vi "2.0.0_BEMF_Calibration.vi"(7 "Data in":T2, 8 "error in (no error)":errorcluster, 9 "AllControls In":T1, 10 "?":T3, 11 "Message Queue out":T4) -> (0 "error out":errorcluster, 1 "Flow":string, 2 "Data":T3, 3 "Message Queue Out":T4, 5 "Data out":T2)   [LabVIEW 2017]
uses:
  Depends/AMC/subVIs/TypeDefs/amc_Message Queue.ctl
  Depends/AMC/subVIs/TypeDefs/amc_Message.ctl
  Depends/Tools/Keyed Array/Tools_KeyedArray KeyedArray.ctl
  Ctrls/Data.ctl
  Ctrls/CSV_Data.ctl
  Ctrls/AllControls.ctl
  DIPC 692 Daemon API/typdef/calibration.ctl
  Ctrls/AlarmIndex.ctl
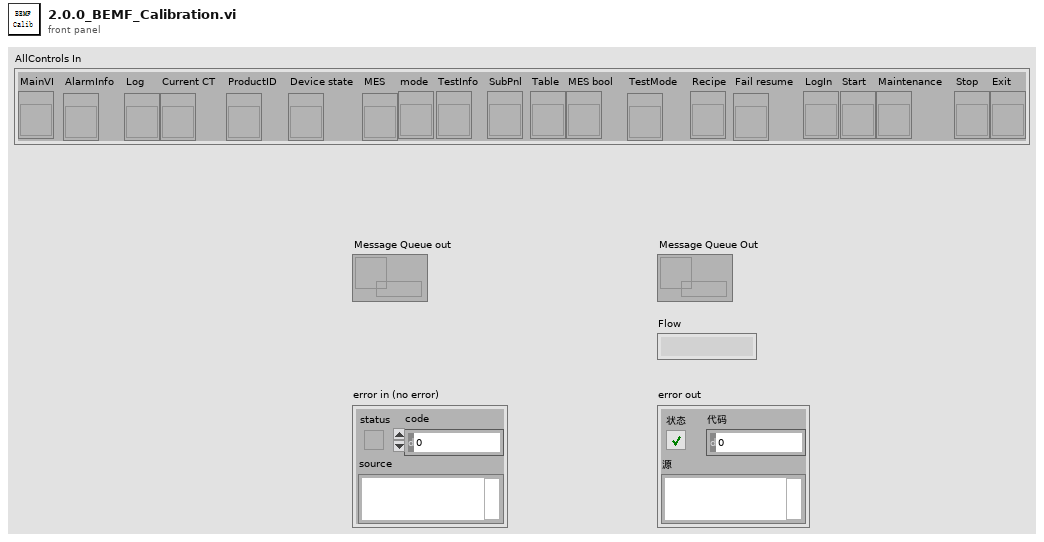
[diagram p1: front panel]
types:
  T1 = typedef "AllControls.ctl" = cluster{"MainVI":refnum<vi>, "AlarmInfo":refnum<vi>, "Log":refnum<vi>, "Current CT":refnum<vi>, "ProductID":refnum<vi>, "Device state":refnum<vi>, "MES":refnum<vi>, "mode":refnum<vi>, "TestInfo":refnum<vi>, "SubPnl":refnum<vi>, "Table":refnum<vi>, "MES bool":refnum<vi>, "TestMode":refnum<vi>, "Recipe":refnum<vi>, "Fail resume":refnum<vi>, "LogIn":refnum<vi>, "Start":refnum<vi>, "Maintenance":refnum<vi>, "Stop":refnum<vi>, "Exit":refnum<vi>}
  T2 = typedef "CSV_Data.ctl" = cluster{"Initialisation":cluster{"LMT - Connect UUT (con COM)":string, "LMT - Software Version (rrel)":string, "LMT - Write SKU file (wskuc)":string, "LMT - SKU file name":string, "Connect UUT DDM":string, "Read DDM EOL Timestamp - Mode":string, "Read DDM EOL Timestamp - Timestamp":string, "Read DDM EOL Timestamp - Rig ID":string, "Read DDM EOL Timestamp - Passmark ID":string, "Read DDM EOL Timestamp - Passmark Rev":string, "Software Version before flashing":string, "Read Hardware Serial":string, "UUT DDM SN":string, "Compare DDM SN with MES SN":string, "Backup PCBA Calibration EEPROM Response - CAL":string, "Flash Firmware Version":string, "Check SW Version":string, "Read DDM SW Version after flashing":string, "Set SKU Config":string, "Ready Status":string, "Set Device Mode to EOL":string, "DDM Parameter - Voltage":string, "DDM Parameter - Current":string, "DDM Parameter - Power":string, "DDM Parameter - Speed":string, "DDM Parameter - Pressure":string, "Tester Parameter - Voltage":string, "Tester Parameter - Current":string, "Tester Parameter - Power":string, "Tester Parameter - Ambient Pressure":string, "Tester Parameter - Ambient Temperature":string, "Calculated Parameter - DDM Pressure Corrected":string, "Calculated Parameter - DDM Real Power":string, "Calculated Parameter - Delta V":string}, "BEMF_Calibration":cluster{"Calibration Result - eol_cold_bemf_temp":string, "DDM Ambient Temp":string, "Restriction Plate Diameter":string, "Calibration Result - eol_bemf_mp_cold_coef_a":string, "Calibration Result - eol_bemf_mp_cold_coef_b":string, "Calibration Result - eol_bemf_mp_cold_coef_c":string, "Calibration Result - eol_bemf_lsi_cold_ref_coeffs":string, "Get - Calibration Result - eol_bemf_lsi_speed":string, "Get - Calibration Result - eol_bemf_lsi_integral_0":string, "Calibration Result - eol_bemf_lsi_integral_1":string, "Get - Calibration Result - eol_bemf_lsi_integral_2":string, "Get - Calibration Result - eol_cold_bemf":string, "Get - Calibration Result - eol_cold_bemf_fisf":string, "Finalise Calibration":string, "Compare -Calibration Result - eol_cold_bemf":string, "Compare -Calibration Result - eol_cold_bemf_fisf":string}, "ECO":cluster{"Reset Power Tune":string, "Reset BEMF FISF Calibration":string, "Restriction Plate Diameter":string, "ECO - Stabilisation Time":string, "ECO - DDM Parameter - Voltage":string, "ECO - DDM Parameter - Current":string, "ECO - DDM Parameter - Power":string, "ECO - DDM Parameter - Measured Power":string, "ECO - DDM Parameter - Speed":string, "ECO - DDM Parameter - Pressure":string, "ECO - Tester Parameter - Voltage":string, "ECO - Tester Parameter - Current":string, "ECO - Tester Parameter - Power":string, "ECO - Tester Parameter - Ambient Pressure":string, "ECO - Tester Parameter - Ambient Temperature":string, "ECO - Tester Parameter - Ambient Humidity":string, "ECO - Calculated Parameter - DDM Pressure Corrected":string, "ECO - Calculated Parameter - DDM Real Power":string, "ECO - Calculated Parameter - Delta V":string, "ECO - Calculated Parameter - Flowrate":string, "ECO - Calculated Parameter - Airwatt":string, "ECO - Formula":string, "PT ECO - Power Tune Mode Status":string}, "BOOST":cluster{"Restriction Plate Diameter":string, "BOOST - Stabilisation Time":string, "BOOST - DDM Parameter - Voltage":string, "BOOST - DDM Parameter - Current":string, "BOOST - DDM Parameter - Power":string, "BOOST - DDM Parameter - Measured Power":string, "BOOST - DDM Parameter - Speed":string, "BOOST - DDM Parameter - Pressure":string, "BOOST - Tester Parameter - Voltage":string, "BOOST - Tester Parameter - Current":string, "BOOST - Tester Parameter - Power":string, "BOOST - Tester Parameter - Ambient Pressure":string, "BOOST - Tester Parameter - Ambient Temperature":string, "BOOST - Tester Parameter - Ambient Humidity":string, "BOOST - Calculated Parameter - DDM Pressure Corrected":string, "BOOST - Calculated Parameter - DDM Real Power":string, "BOOST - Calculated Parameter - Delta V":string, "BOOST - Calculated Parameter - Flowrate":string, "BOOST - Calculated Parameter - Airwatt":string, "BOOST - Get AM Presence":string, "Air Muscle Turn Off Status":string, "BOOST - Air Muscle Calculated Parameter - Airwatt B":string, "BOOST - Air Muscle Calculate Airwatt Delta":string, "PT BOOST - Power Tune Mode Status":string, "Finalise Calibration":string, "ECO - Get AW Calibration value":string, "BOOST - Get AW Calibration value":string}, "MAX":cluster{"Restriction Plate Diameter":string, "MAX - Stabilisation Time":string, "Get Average Delta Tmag (LSIdelta_FISFdelta_LSItmag_FISFtmag_IIRtmag)":string, "Get Average Delta Tmag FISF":string, "MAX - DDM Parameter - Voltage":string, "MAX - DDM Parameter - Current":string, "MAX - DDM Parameter - Power":string, "MAX - DDM Parameter - Measured Power":string, "MAX - DDM Parameter - Speed":string, "MAX - DDM Parameter - Pressure":string, "MAX - Tester Parameter - Voltage":string, "MAX - Tester Parameter - Current":string, "MAX - Tester Parameter - Power":string, "MAX - Tester Parameter - Ambient Pressure":string, "MAX - Tester Parameter - Ambient Temperature":string, "MAX - Tester Parameter - Ambient Humidity":string, "MAX - Calculated Parameter - DDM Pressure Corrected":string, "MAX - Calculated Parameter - DDM Real Power":string, "MAX - Calculated Parameter - Delta V":string, "MAX - Calculated Parameter - Flowrate":string, "MAX - Calculated Parameter - Airwatt":string, "MAX_FISF_Check_Average_Delta_Tmag":string, "MAX - FISF - BEMF Finetune Result":string, "MAX tune - Delta P1":string, "MAX tune - Calculated Parameter - Airwatt":string, "Calculate Delta Airwatts - MAX finetune - Delta P2":string, "MAX finetune - DDM Parameter - Voltage":string, "MAX finetune - DDM Parameter - Current":string, "MAX finetune - DDM Parameter - Power":string, "MAX finetune - DDM Parameter - Measured Power":string, "MAX finetune - DDM Parameter - Speed":string, "MAX finetune - DDM Parameter - Pressure":string, "MAX finetune - Tester Parameter - Voltage":string, "MAX finetune - Tester Parameter - Current":string, "MAX finetune - Tester Parameter - Power":string, "MAX finetune - Tester Parameter - Ambient Pressure":string, "MAX finetune - Tester Parameter - Ambient Temperature":string, "MAX finetune - Tester Parameter - Ambient Humidity":string, "MAX finetune - Calculated Parameter - DDM Pressure Corrected":string, "MAX finetune - Calculated Parameter - DDM Real Power":string, "MAX finetune - Calculated Parameter - Delta V":string, "MAX finetune - Calculated Parameter - Flowrate":string, "MAX finetune - Calculated Parameter - Airwatt":string, "Check Derate Result":string, "Delta Tmag FISF":string, "Get Hot BEMF Result":string, "Calculate delta Pressure":string, "Finalise Calibration":string, "Calculate & Check Delta BEMF":string, "Delta P Airwatts Value":string}, "LL":cluster{"DDM Ambient Temp":string, "Restriction Plate Diameter":string, "LL - DDM Parameter - Voltage":string, "LL - DDM Parameter - Current":string, "LL - DDM Parameter - Power":string, "LL - DDM Parameter - Measured Power":string, "LL - DDM Parameter - Speed":string, "LL - DDM Parameter - Pressure":string, "LL - Tester Parameter - Voltage":string, "LL - Tester Parameter - Current":string, "LL - Tester Parameter - Power":string, "LL - DDM Real Power":string, "LL - Calibrate Task Detect LL":string}, "HL":cluster{"HL - DDM Parameter - Voltage":string, "HL - DDM Parameter - Current":string, "HL - DDM Parameter - Power":string, "HL - DDM Parameter - Measured Power":string, "HL - DDM Parameter - Speed":string, "HL - DDM Parameter - Pressure":string, "HL - Tester Parameter - Voltage":string, "HL - Tester Parameter - Current":string, "HL - Tester Parameter - Power":string, "HL - DDM Real Power":string, "HL - Calibrate Task Detect HL":string}, "LH":cluster{"Restriction Plate Diameter":string, "LH - DDM Parameter - Voltage":string, "LH - DDM Parameter - Current":string, "LH - DDM Parameter - Power":string, "LH - DDM Parameter - Measured Power":string, "LH - DDM Parameter - Speed":string, "LH - DDM Parameter - Pressure":string, "LH - Tester Parameter - Voltage":string, "LH - Tester Parameter - Current":string, "LH - Tester Parameter - Power":string, "LH - DDM Real Power":string, "LH - Calibrate Task Detect LH":string}, "HH":cluster{"HH - DDM Parameter - Voltage":string, "HH - DDM Parameter - Current":string, "HH - DDM Parameter - Power":string, "HH - DDM Parameter - Measured Power":string, "HH - DDM Parameter - Speed":string, "HH - DDM Parameter - Pressure":string, "HH - Tester Parameter - Voltage":string, "HH - Tester Parameter - Current":string, "HH - Tester Parameter - Power":string, "HH - DDM Real Power":string, "HH - Calibrate Task Detect HH":string}, "Inlet Blockage Calibration":cluster{"Inlet Blockage Calibration - DDM Parameter - Voltage":string, "Inlet Blockage Calibration - DDM Parameter - Current":string, "Inlet Blockage Calibration - DDM Parameter - Power":string, "Inlet Blockage Calibration - DDM Parameter - Measured Power":string, "Inlet Blockage Calibration - DDM Parameter - Speed":string, "Inlet Blockage Calibration - DDM Parameter - Pressure":string, "Inlet Blockage Calibration - Tester Parameter - Voltage":string, "Inlet Blockage Calibration - Tester Parameter - Current":string, "Inlet Blockage Calibration - Tester Parameter - Power":string, "Inlet Blockage Calibration - DDM Real Power":string, "Calibration Inlet Blockage_E":string, "Finalise Calibration":string, "Get Task Detect LL":string, "Get Task Detect HL":string, "Get Task Detect LH":string, "Get Task Detect HH":string, "Calibration Inlet Blockage":string, "Calibration eol cold bemf temp":string}, "GOOD":cluster{"GOOD UNIT - Clear EEPROM Error Log":string, "GOOD UNIT - Write Product Timestamp - Mode":string, "GOOD UNIT - Write Product Timestamp - Timestamp":string, "GOOD UNIT - Write Product Timestamp - Rig ID":string, "GOOD UNIT - Write Product Timestamp - Passmark ID":string, "GOOD UNIT - Write Product Timestamp - Passmark Rev":string, "GOOD UNIT - Set Device Mode to PROD":string, "GOOD UNIT - Backup PCBA Calibration EEPROM Response":string, "GOOD UNIT - Check Security Bit":string, "GOOD UNIT - Set Calibration Lock":string, "GOOD UNIT - Get_Calibration_Lock":string, "GOOD UNIT - Disconnect UUT":string}, "NG":cluster{"NG UNIT - Read NVM Error":string, "NG UNIT - Set Device Mode to FCT":string, "NG UNIT - Backup PCBA Calibration EEPROM Response - CAL":string, "NG UNIT - Backup PCBA Calibration EEPROM Response - ERROR":string, "NG UNIT - Backup PCBA Calibration EEPROM Response - USAGE":string, "NG UNIT - Disconnect UUT":string}, "SN":string, "Table":string[][], "Count":cluster{"Total":i32, "OK":i32, "NG":i32, "Yield":dbl}, "Start Time":timestamp, "daemon reference":refnum<k5>, "CT":dbl, "Config":string[][], "OK/NG":bool, "Station ID":string, "MES DDM SN":string, "MES PCBA SN":string, "Retest":string, "UID":string, "Initialisation_Status":cluster{"LMT - Connect UUT (con COM)":string, "LMT - Software Version (rrel)":string, "LMT - Write SKU file (wskuc)":string, "LMT - SKU file name":string, "Connect UUT DDM":string, "Read DDM EOL Timestamp - Mode":string, "Read DDM EOL Timestamp - Timestamp":string, "Read DDM EOL Timestamp - Rig ID":string, "Read DDM EOL Timestamp - Passmark ID":string, "Read DDM EOL Timestamp - Passmark Rev":string, "Software Version before flashing":string, "Read Hardware Serial":string, "UUT DDM SN":string, "Compare DDM SN with MES SN":string, "Backup PCBA Calibration EEPROM Response - CAL":string, "Flash Firmware Version":string, "Check SW Version":string, "Read DDM SW Version after flashing":string, "Set SKU Config":string, "Ready Status":string, "Set Device Mode to EOL":string, "DDM Parameter - Voltage":string, "DDM Parameter - Current":string, "DDM Parameter - Power":string, "DDM Parameter - Speed":string, "DDM Parameter - Pressure":string, "Tester Parameter - Voltage":string, "Tester Parameter - Current":string, "Tester Parameter - Power":string, "Tester Parameter - Ambient Pressure":string, "Tester Parameter - Ambient Temperature":string, "Calculated Parameter - DDM Pressure Corrected":string, "Calculated Parameter - DDM Real Power":string, "Calculated Parameter - Delta V":string}, "BEMF_Calibration_Status":cluster{"Calibration Result - eol_cold_bemf_temp":string, "DDM Ambient Temp":string, "Restriction Plate Diameter":string, "Calibration Result - eol_bemf_mp_cold_coef_a":string, "Calibration Result - eol_bemf_mp_cold_coef_b":string, "Calibration Result - eol_bemf_mp_cold_coef_c":string, "Calibration Result - eol_bemf_lsi_cold_ref_coeffs":string, "Get - Calibration Result - eol_bemf_lsi_speed":string, "Get - Calibration Result - eol_bemf_lsi_integral_0":string, "Calibration Result - eol_bemf_lsi_integral_1":string, "Get - Calibration Result - eol_bemf_lsi_integral_2":string, "Get - Calibration Result - eol_cold_bemf":string, "Get - Calibration Result - eol_cold_bemf_fisf":string, "Finalise Calibration":string, "Compare -Calibration Result - eol_cold_bemf":string, "Compare -Calibration Result - eol_cold_bemf_fisf":string}, "ECO_Status":cluster{"Reset Power Tune":string, "Reset BEMF FISF Calibration":string, "Restriction Plate Diameter":string, "ECO - Stabilisation Time":string, "ECO - DDM Parameter - Voltage":string, "ECO - DDM Parameter - Current":string, "ECO - DDM Parameter - Power":string, "ECO - DDM Parameter - Measured Power":string, "ECO - DDM Parameter - Speed":string, "ECO - DDM Parameter - Pressure":string, "ECO - Tester Parameter - Voltage":string, "ECO - Tester Parameter - Current":string, "ECO - Tester Parameter - Power":string, "ECO - Tester Parameter - Ambient Pressure":string, "ECO - Tester Parameter - Ambient Temperature":string, "ECO - Tester Parameter - Ambient Humidity":string, "ECO - Calculated Parameter - DDM Pressure Corrected":string, "ECO - Calculated Parameter - DDM Real Power":string, "ECO - Calculated Parameter - Delta V":string, "ECO - Calculated Parameter - Flowrate":string, "ECO - Calculated Parameter - Airwatt":string, "ECO - Formula":string, "PT ECO - Power Tune Mode Status":string}, "BOOST_Status":cluster{"Restriction Plate Diameter":string, "BOOST - Stabilisation Time":string, "BOOST - DDM Parameter - Voltage":string, "BOOST - DDM Parameter - Current":string, "BOOST - DDM Parameter - Power":string, "BOOST - DDM Parameter - Measured Power":string, "BOOST - DDM Parameter - Speed":string, "BOOST - DDM Parameter - Pressure":string, "BOOST - Tester Parameter - Voltage":string, "BOOST - Tester Parameter - Current":string, "BOOST - Tester Parameter - Power":string, "BOOST - Tester Parameter - Ambient Pressure":string, "BOOST - Tester Parameter - Ambient Temperature":string, "BOOST - Tester Parameter - Ambient Humidity":string, "BOOST - Calculated Parameter - DDM Pressure Corrected":string, "BOOST - Calculated Parameter - DDM Real Power":string, "BOOST - Calculated Parameter - Delta V":string, "BOOST - Calculated Parameter - Flowrate":string, "BOOST - Calculated Parameter - Airwatt":string, "BOOST - Get AM Presence":string, "Air Muscle Turn Off Status":string, "BOOST - Air Muscle Calculated Parameter - Airwatt B":string, "BOOST - Air Muscle Calculate Airwatt Delta":string, "PT BOOST - Power Tune Mode Status":string, "Finalise Calibration":string, "ECO - Get AW Calibration value":string, "BOOST - Get AW Calibration value":string}, "MAX_Status":cluster{"Restriction Plate Diameter":string, "MAX - Stabilisation Time":string, "Get Average Delta Tmag (LSIdelta_FISFdelta_LSItmag_FISFtmag_IIRtmag)":string, "Get Average Delta Tmag FISF":string, "MAX - DDM Parameter - Voltage":string, "MAX - DDM Parameter - Current":string, "MAX - DDM Parameter - Power":string, "MAX - DDM Parameter - Measured Power":string, "MAX - DDM Parameter - Speed":string, "MAX - DDM Parameter - Pressure":string, "MAX - Tester Parameter - Voltage":string, "MAX - Tester Parameter - Current":string, "MAX - Tester Parameter - Power":string, "MAX - Tester Parameter - Ambient Pressure":string, "MAX - Tester Parameter - Ambient Temperature":string, "MAX - Tester Parameter - Ambient Humidity":string, "MAX - Calculated Parameter - DDM Pressure Corrected":string, "MAX - Calculated Parameter - DDM Real Power":string, "MAX - Calculated Parameter - Delta V":string, "MAX - Calculated Parameter - Flowrate":string, "MAX - Calculated Parameter - Airwatt":string, "MAX_FISF_Check_Average_Delta_Tmag":string, "MAX - FISF - BEMF Finetune Result":string, "MAX tune - Delta P1":string, "MAX tune - Calculated Parameter - Airwatt":string, "Calculate Delta Airwatts - MAX finetune - Delta P2":string, "MAX finetune - DDM Parameter - Voltage":string, "MAX finetune - DDM Parameter - Current":string, "MAX finetune - DDM Parameter - Power":string, "MAX finetune - DDM Parameter - Measured Power":string, "MAX finetune - DDM Parameter - Speed":string, "MAX finetune - DDM Parameter - Pressure":string, "MAX finetune - Tester Parameter - Voltage":string, "MAX finetune - Tester Parameter - Current":string, "MAX finetune - Tester Parameter - Power":string, "MAX finetune - Tester Parameter - Ambient Pressure":string, "MAX finetune - Tester Parameter - Ambient Temperature":string, "MAX finetune - Tester Parameter - Ambient Humidity":string, "MAX finetune - Calculated Parameter - DDM Pressure Corrected":string, "MAX finetune - Calculated Parameter - DDM Real Power":string, "MAX finetune - Calculated Parameter - Delta V":string, "MAX finetune - Calculated Parameter - Flowrate":string, "MAX finetune - Calculated Parameter - Airwatt":string, "Check Derate Result":string, "Delta Tmag FISF":string, "Get Hot BEMF Result":string, "Calculate delta Pressure":string, "Finalise Calibration":string, "Calculate & Check Delta BEMF":string, "Delta P Airwatts Value":string}, "LL_Status":cluster{"DDM Ambient Temp":string, "Restriction Plate Diameter":string, "LL - DDM Parameter - Voltage":string, "LL - DDM Parameter - Current":string, "LL - DDM Parameter - Power":string, "LL - DDM Parameter - Measured Power":string, "LL - DDM Parameter - Speed":string, "LL - DDM Parameter - Pressure":string, "LL - Tester Parameter - Voltage":string, "LL - Tester Parameter - Current":string, "LL - Tester Parameter - Power":string, "LL - DDM Real Power":string, "LL - Calibrate Task Detect LL":string}, "HL_Status":cluster{"HL - DDM Parameter - Voltage":string, "HL - DDM Parameter - Current":string, "HL - DDM Parameter - Power":string, "HL - DDM Parameter - Measured Power":string, "HL - DDM Parameter - Speed":string, "HL - DDM Parameter - Pressure":string, "HL - Tester Parameter - Voltage":string, "HL - Tester Parameter - Current":string, "HL - Tester Parameter - Power":string, "HL - DDM Real Power":string, "HL - Calibrate Task Detect HL":string}, "LH_Status":cluster{"Restriction Plate Diameter":string, "LH - DDM Parameter - Voltage":string, "LH - DDM Parameter - Current":string, "LH - DDM Parameter - Power":string, "LH - DDM Parameter - Measured Power":string, "LH - DDM Parameter - Speed":string, "LH - DDM Parameter - Pressure":string, "LH - Tester Parameter - Voltage":string, "LH - Tester Parameter - Current":string, "LH - Tester Parameter - Power":string, "LH - DDM Real Power":string, "LH - Calibrate Task Detect LH":string}, "HH_Status":cluster{"HH - DDM Parameter - Voltage":string, "HH - DDM Parameter - Current":string, "HH - DDM Parameter - Power":string, "HH - DDM Parameter - Measured Power":string, "HH - DDM Parameter - Speed":string, "HH - DDM Parameter - Pressure":string, "HH - Tester Parameter - Voltage":string, "HH - Tester Parameter - Current":string, "HH - Tester Parameter - Power":string, "HH - DDM Real Power":string, "HH - Calibrate Task Detect HH":string}, "Inlet Blockage Calibration_Status":cluster{"Inlet Blockage Calibration - DDM Parameter - Voltage":string, "Inlet Blockage Calibration - DDM Parameter - Current":string, "Inlet Blockage Calibration - DDM Parameter - Power":string, "Inlet Blockage Calibration - DDM Parameter - Measured Power":string, "Inlet Blockage Calibration - DDM Parameter - Speed":string, "Inlet Blockage Calibration - DDM Parameter - Pressure":string, "Inlet Blockage Calibration - Tester Parameter - Voltage":string, "Inlet Blockage Calibration - Tester Parameter - Current":string, "Inlet Blockage Calibration - Tester Parameter - Power":string, "Inlet Blockage Calibration - DDM Real Power":string, "Calibration Inlet Blockage_E":string, "Finalise Calibration":string, "Get Task Detect LL":string, "Get Task Detect HL":string, "Get Task Detect LH":string, "Get Task Detect HH":string, "Calibration Inlet Blockage":string, "Calibration eol cold bemf temp":string}, "GOOD_Status":cluster{"GOOD UNIT - Clear EEPROM Error Log":string, "GOOD UNIT - Write Product Timestamp - Mode":string, "GOOD UNIT - Write Product Timestamp - Timestamp":string, "GOOD UNIT - Write Product Timestamp - Rig ID":string, "GOOD UNIT - Write Product Timestamp - Passmark ID":string, "GOOD UNIT - Write Product Timestamp - Passmark Rev":string, "GOOD UNIT - Set Device Mode to PROD":string, "GOOD UNIT - Backup PCBA Calibration EEPROM Response":string, "GOOD UNIT - Check Security Bit":string, "GOOD UNIT - Set Calibration Lock":string, "GOOD UNIT - Get_Calibration_Lock":string, "GOOD UNIT - Disconnect UUT":string}, "NG_Status":cluster{"NG UNIT - Read NVM Error":string, "NG UNIT - Set Device Mode to FCT":string, "NG UNIT - Backup PCBA Calibration EEPROM Response - CAL":string, "NG UNIT - Backup PCBA Calibration EEPROM Response - ERROR":string, "NG UNIT - Backup PCBA Calibration EEPROM Response - USAGE":string, "NG UNIT - Disconnect UUT":string}, "SKU":string, "Plate_Diameter":string, "Alarm":string}
  T3 = typedef "Data.ctl" = cluster{"Initialisation":cluster{"DDM_Parameter":dbl[], "DDM_Parameter_status":bool[], "Get_Tester_Parameter":dbl[], "Get_Tester_Parameter_status":bool[], "Cal_Tester_Parameter":dbl[], "Cal_Tester_Parameter_status":bool[], "sw_version_before_status":bool, "sw_version_after_status":bool, "Set_SKU_Config_With_LMT_status":bool, "FCT_timestamp_status":bool, "LMT_Connect_to_UUT_status":bool}, "BEMF_Calibration":cluster{"Read_ambient_temperature":dbl, "Calibration_Vaule":dbl[], "Calibration_Vaule _B":dbl[], "Calibration_Vaule_status":bool[], "Calibration_Vaule_B_status":bool[]}, "ECO":cluster{"DDM_Parameter":dbl[], "DDM_Parameter_status":bool[], "Get_Tester_Parameter":dbl[], "Get_Tester_Parameter_status":bool[], "Cal_Tester_Parameter":dbl[], "Cal_Tester_Parameter_status":bool[], "DDM_Parameter_after_power_tune":dbl[], "Get_Tester_Parameter_after_power_tune":dbl[], "Cal_Tester_Parameter_after_power_tune":dbl[], "Cal_Tester_Parameter_after_power_tune_status":bool[], "Delta_P":dbl}, "BOOST":cluster{"DDM_Parameter":dbl[], "DDM_Parameter_status":bool[], "Get_Tester_Parameter":dbl[], "Get_Tester_Parameter_status":bool[], "Cal_Tester_Parameter":dbl[], "Cal_Tester_Parameter_status":bool[], "DDM_Parameter_after_power_tune":dbl[], "Get_Tester_Parameter_after_power_tune":dbl[], "Cal_Tester_Parameter_after_power_tune":dbl[], "Cal_Tester_Parameter_after_power_tune_status":bool[], "airwatts_am_off":dbl, "AW_Delta_(AM_on_and_off)":dbl, "AW_Delta_(AM_on_and_off)_Status":bool, "Delta_P":dbl}, "MAX":cluster{"Average_Tmag_Data":cluster{"LSI Delta in degC":dbl, "FISF Delta in degc":dbl, "LSI Tmag in degC":dbl, "Fisf Tmag in degC":dbl, "IIR Tmag in degC":dbl}, "DDM_Parameter":dbl[], "DDM_Parameter_status":bool[], "Get_Tester_Parameter":dbl[], "Get_Tester_Parameter_status":bool[], "Cal_Tester_Parameter":dbl[], "BEMF_Finetune":cluster{"eol_bemf_mp_cold_coef_c":dbl, "eol_cold_bemf_fisf_offset":dbl}, "AW_Tune":cluster{"delta_P1":dbl, "delta_P_Setting":dbl}, "DDM_Parameter_after_Airwatts_Tune":dbl[], "Get_Tester_Parameter_after_Airwatts_Tune":dbl[], "Cal_Tester_Parameter_after_Airwatts_Tune":dbl[], "DDM_Parameter_after_Airwatts_Finetune":dbl[], "Get_Tester_Parameter_after_Airwatts_Finetune":dbl[], "Cal_Tester_Parameter_after_Airwatts_Finetune":dbl[], "AW_Finetune":cluster{"delta_P2":dbl, "delta_P_Setting":dbl}, "Delta_Tmag_after_tune":cluster{"LSI Delta in degC":dbl, "FISF Delta in degc":dbl, "LSI Tmag in degC":dbl, "Fisf Tmag in degC":dbl, "IIR Tmag in degC":dbl}, "Hot Bemf in mV":dbl, "DDM_Pressure":dbl, "Delta_Pressure":dbl, " Cold Bemf in mV":dbl, " delta Bemf":dbl, " delta p":dbl, "Delta_Pressure_status":bool, " delta Bemf_status":bool, "LSI Delta in degC_status":bool, "FISF Delta in degc_status":bool, "Max_check_derate_status_status":bool, "Average_All_data":dbl[][], "Average_Tmag_Data_status":bool[], "Average_Tmag_Data_after_tune_status":bool[], "Cal_Tester_Parameter_status":bool[], "Cal_Tester_Parameter_status_after_Airwatts_Tune":bool[], "Cal_Tester_Parameter_status_after_Airwatts_FineTune":bool[]}, "Task_Detect_Calib":cluster{"LL":cluster{"DDM_Parameter":dbl[], "DDM_Parameter_status":bool[], "Get_Tester_Parameter":dbl[], "Get_Tester_Parameter_status":bool[], "Set_task_detect_A":dbl, "Set_task_detect_A_Status":bool}, "HL":cluster{"DDM_Parameter":dbl[], "DDM_Parameter_status":bool[], "Get_Tester_Parameter":dbl[], "Get_Tester_Parameter_status":bool[], "Set_task_detect_B":dbl, "Set_task_detect_B_Status":bool}, "LH":cluster{"DDM_Parameter":dbl[], "DDM_Parameter_status":bool[], "Get_Tester_Parameter":dbl[], "Get_Tester_Parameter_status":bool[], "Set_task_detect_C":dbl, "Set_task_detect_C_Status":bool}, "HH":cluster{"DDM_Parameter":dbl[], "DDM_Parameter_status":bool[], "Get_Tester_Parameter":dbl[], "Get_Tester_Parameter_status":bool[], "Set_task_detect_D":dbl, "Read_and_check_calibration_Status":bool[], "Set_task_detect_D_Status":bool}, "Get_eol_inlet_blockage_E":dbl, "Calib_vaule":cluster{"Get_task_detect_LL":dbl, "Get_task_detect_HL":dbl, "Get_task_detect_LH":dbl, "Get_task_detect_HH":dbl, "eol_inlet_blockage":dbl, "eol_code_bemf_temp":dbl}, "calibrated temp":dbl, "Inlet_Blockage_Calibration":cluster{"DDM_Parameter":dbl[], "DDM_Parameter_status":bool[], "Get_Tester_Parameter":dbl[], "Get_Tester_Parameter_status":bool[]}, "Get_eol_inlet_blockage_E_Status":bool}, "good":cluster{"Write_Product_TS":cluster{"TIMESTAMP":i64, "RIG_ID":i64, "PASSMARK_ID":i64, "PASSMARK_REV":i64}, "Read_Product_TS":cluster{"TIMESTAMP":i64, "RIG_ID":i64, "PASSMARK_ID":i64, "PASSMARK_REV":i64}, "Good_Check_Secuity_Bit_Stauts":bool}}
  T4 = typedef "amc_Message Queue.ctl" = refnum<queue>
  T5 = typedef "HD Config.ctl" = cluster{" PC":cluster{"PC Address":u8[], "PC Port":i32}, "FCO":cluster{"COM":refnum<visa-resource-name>, "Baudrate":u32}, "DC Power ":cluster{"COM":refnum<visa-resource-name>, "Baudrate":u32}, "PW3336":cluster{"COM":refnum<visa-resource-name>, "Baudrate":u32}, "Lefoo":cluster{"COM":refnum<visa-resource-name>, "Baudrate":u32}, "AI Model":cluster{"COM":refnum<visa-resource-name>, "Baudrate":u32}, "DIPC":cluster{"COM":refnum<visa-resource-name>}, "RFID":cluster{"IP Address":string, "Port":u16, "Retry":u16}, "Motor":cluster{"COM":refnum<visa-resource-name>, "Baudrate":u32}, "Fail_resume_mode":bool, "GRR":bool}
  T6 = typedef "calibration.ctl" = string
  T7 = typedef "AlarmIndex.ctl" = enum16{"E-Stop", "Safety light grid", "UUT Sealing Cylinder HomePoint", "UUT Sealing Cylinder WorkPoint", "Orifice fixed Cylinder L HomePoint", "Orifice fixed Cylinder L WorkPoint", "Orifice fixed Cylinder R HomePoint", "Orifice fixed Cylinder R WorkPoint", "UUT Cylinder HomePoint", "UUT Cylinder WorkPoint", "Carrier fixed Cylinder L HomePoint", "Carrier fixed Cylinder L WorkPoint", "Carrier fixed Cylinder R HomePoint", "Carrier fixed Cylinder R WorkPoint", "Probe Cylinder HomePoint", "Probe Cylinder WorkPoint", "Motor Error", "Test Error"}
  T8 = typedef "Position Config.ctl" = cluster{"OrificeSize_12.7":i32, "OrificeSize_13":i32, "OrificeSize_30":i32, "OrificeSize_16":i32}
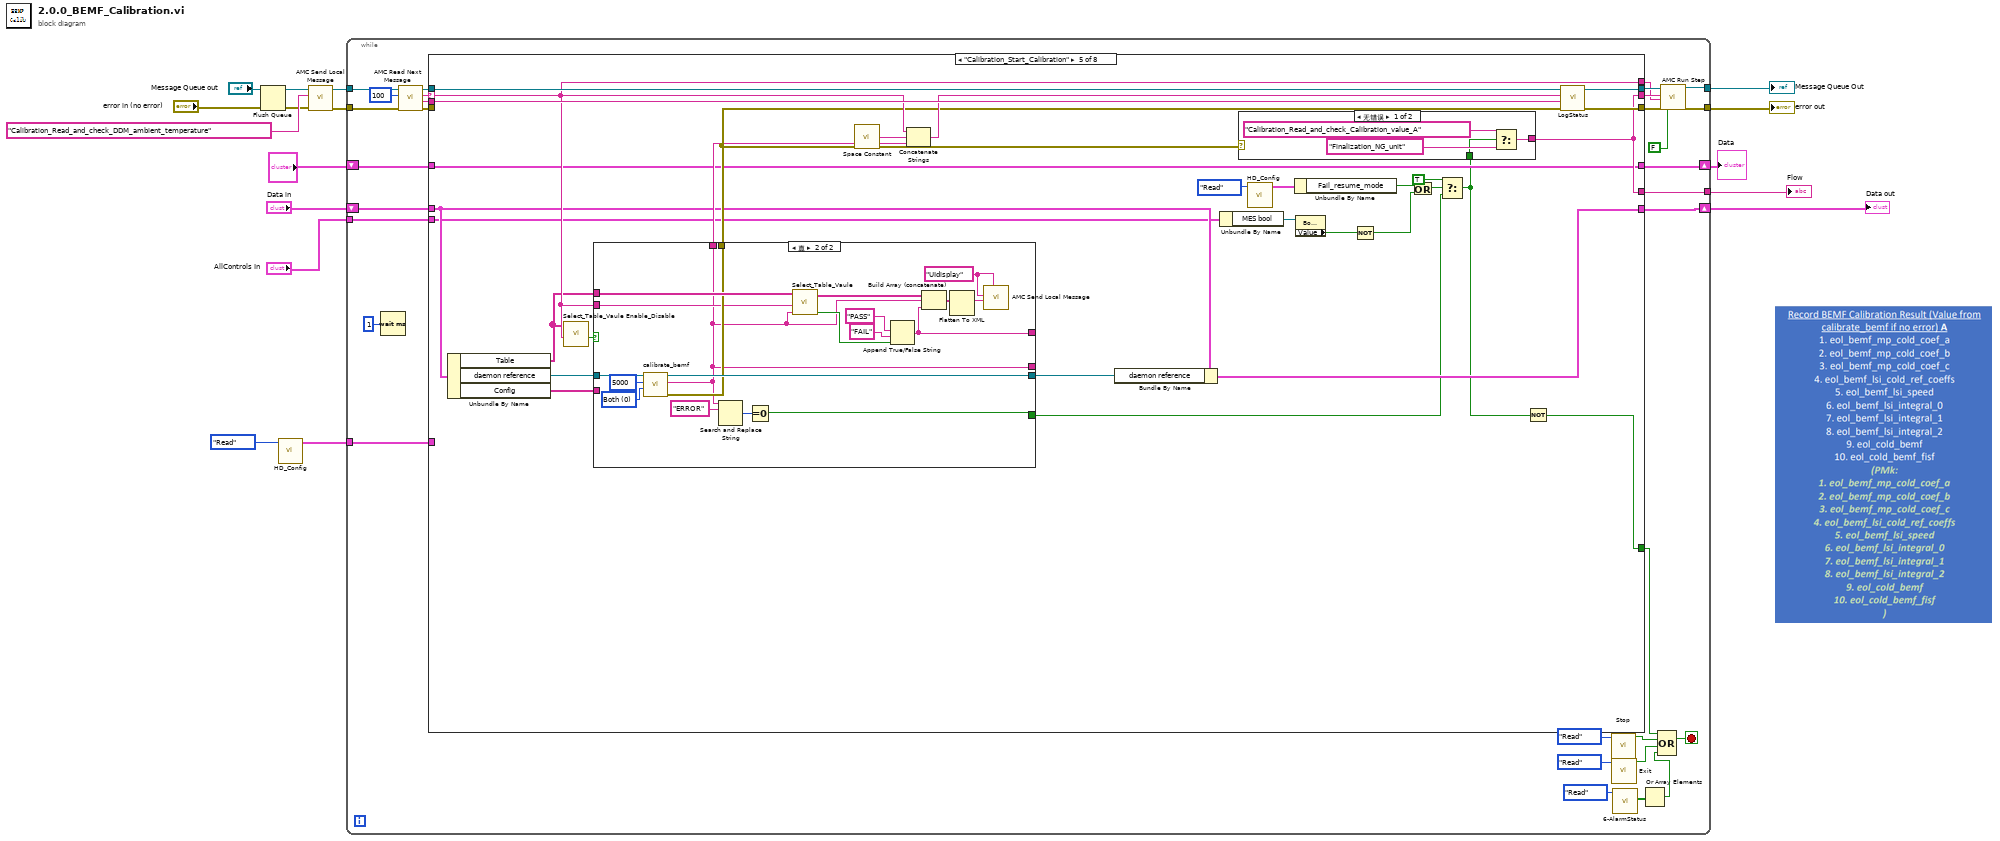
[diagram p0: block diagram]
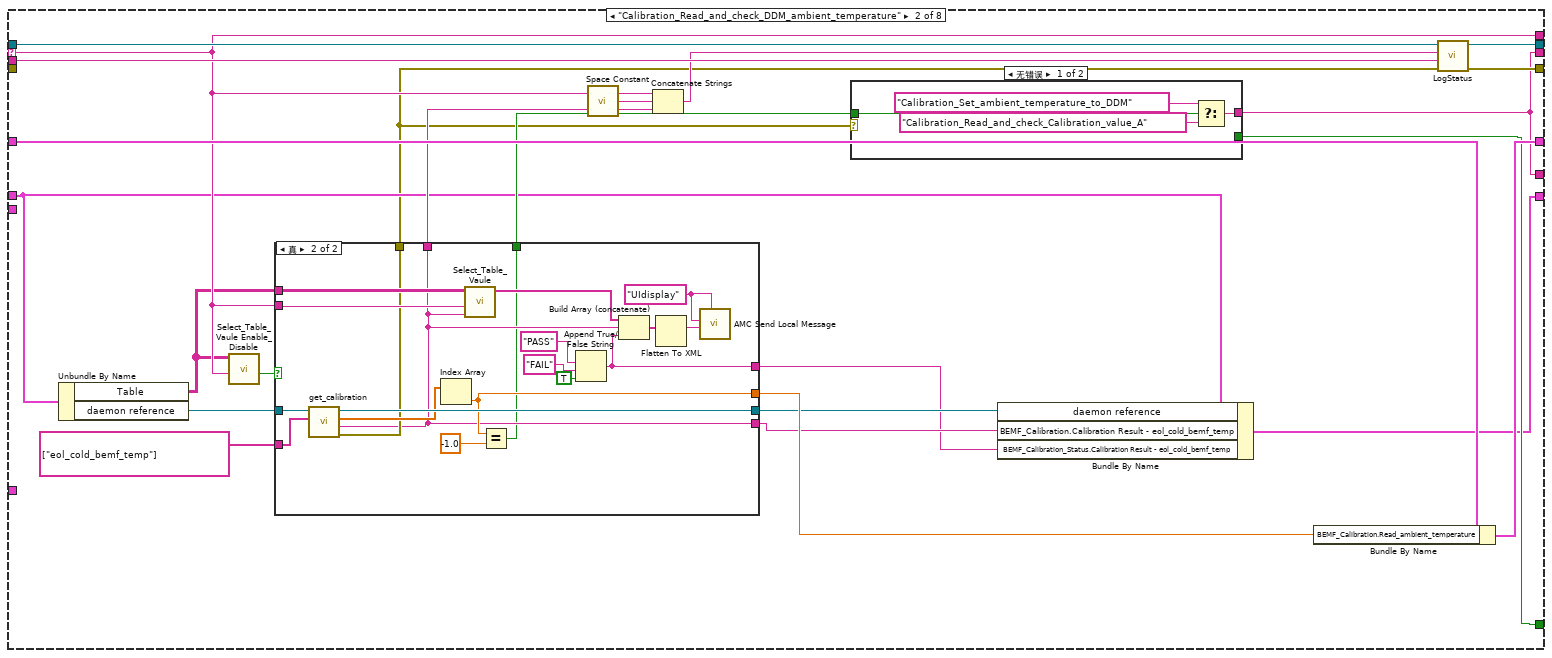
[diagram p3: hidden frame]
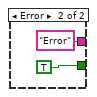
[diagram p4: hidden frame]
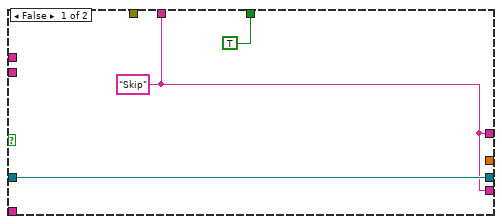
[diagram p5: hidden frame]
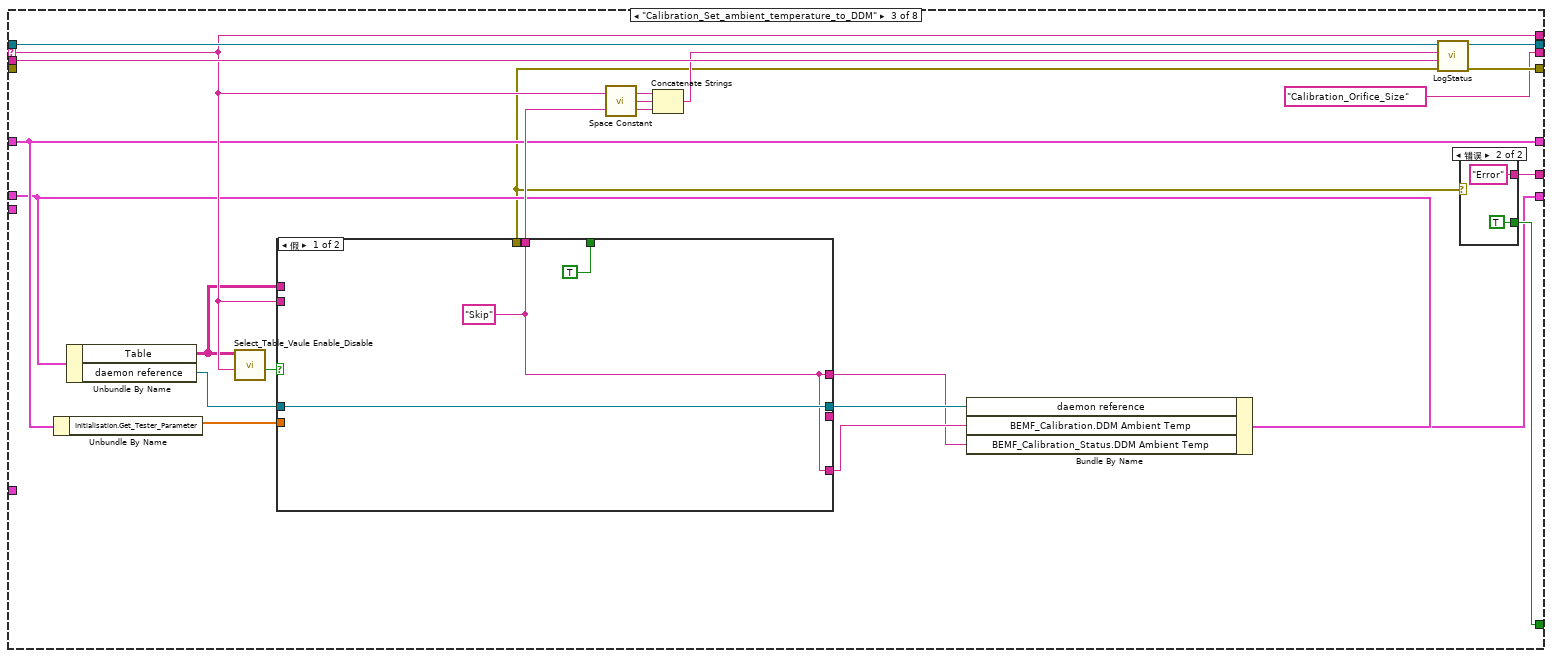
[diagram p6: hidden frame]
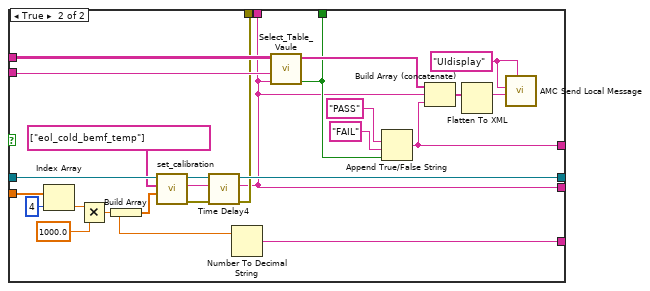
[diagram p8: hidden frame]
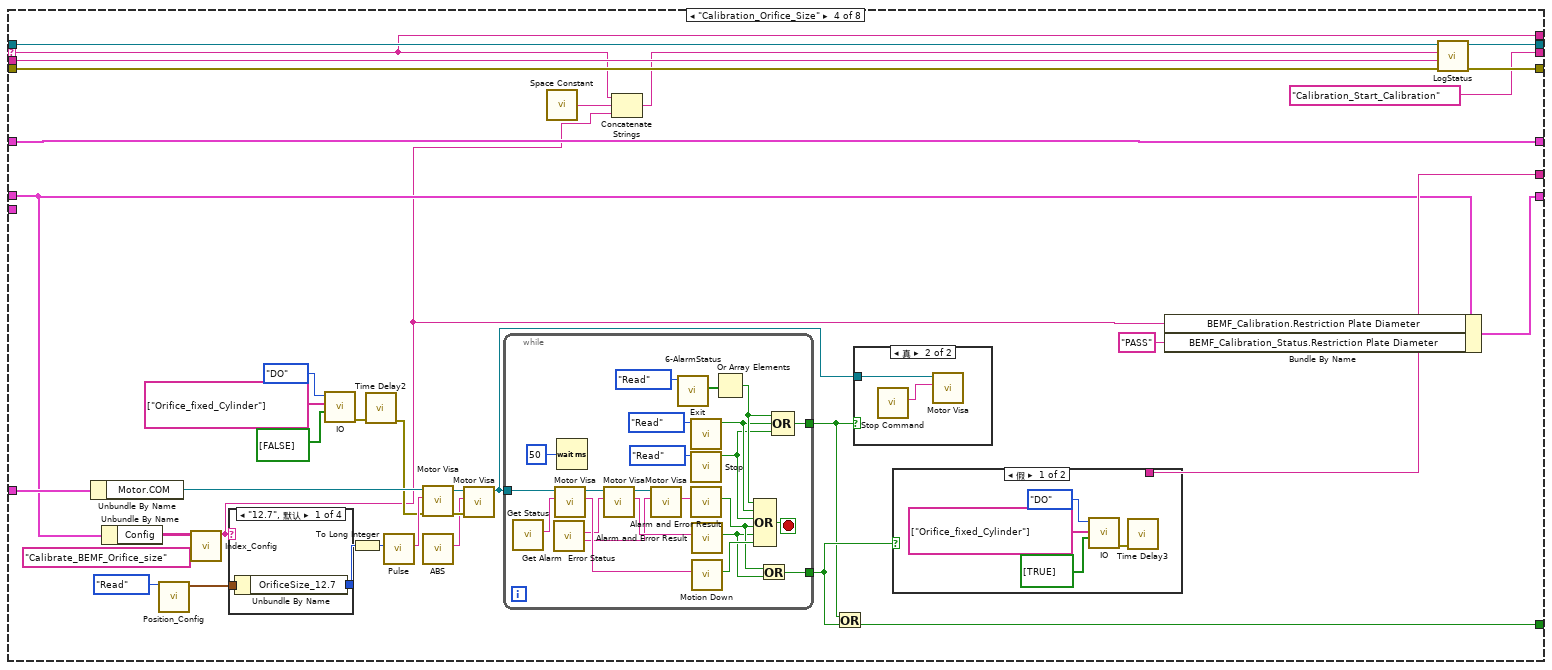
[diagram p9: hidden frame]
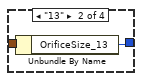
[diagram p11: hidden frame]
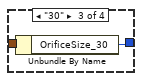
[diagram p12: hidden frame]
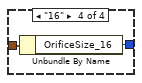
[diagram p13: hidden frame]
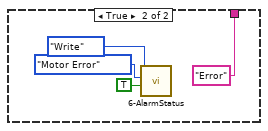
[diagram p14: hidden frame]
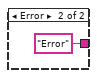
[diagram p15: hidden frame]
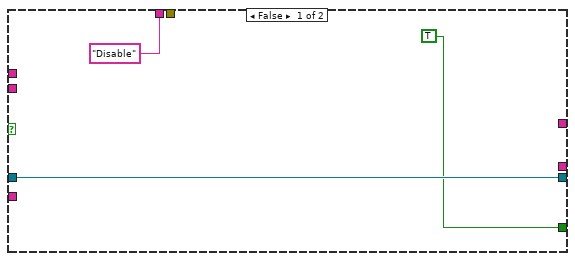
[diagram p16: hidden frame]
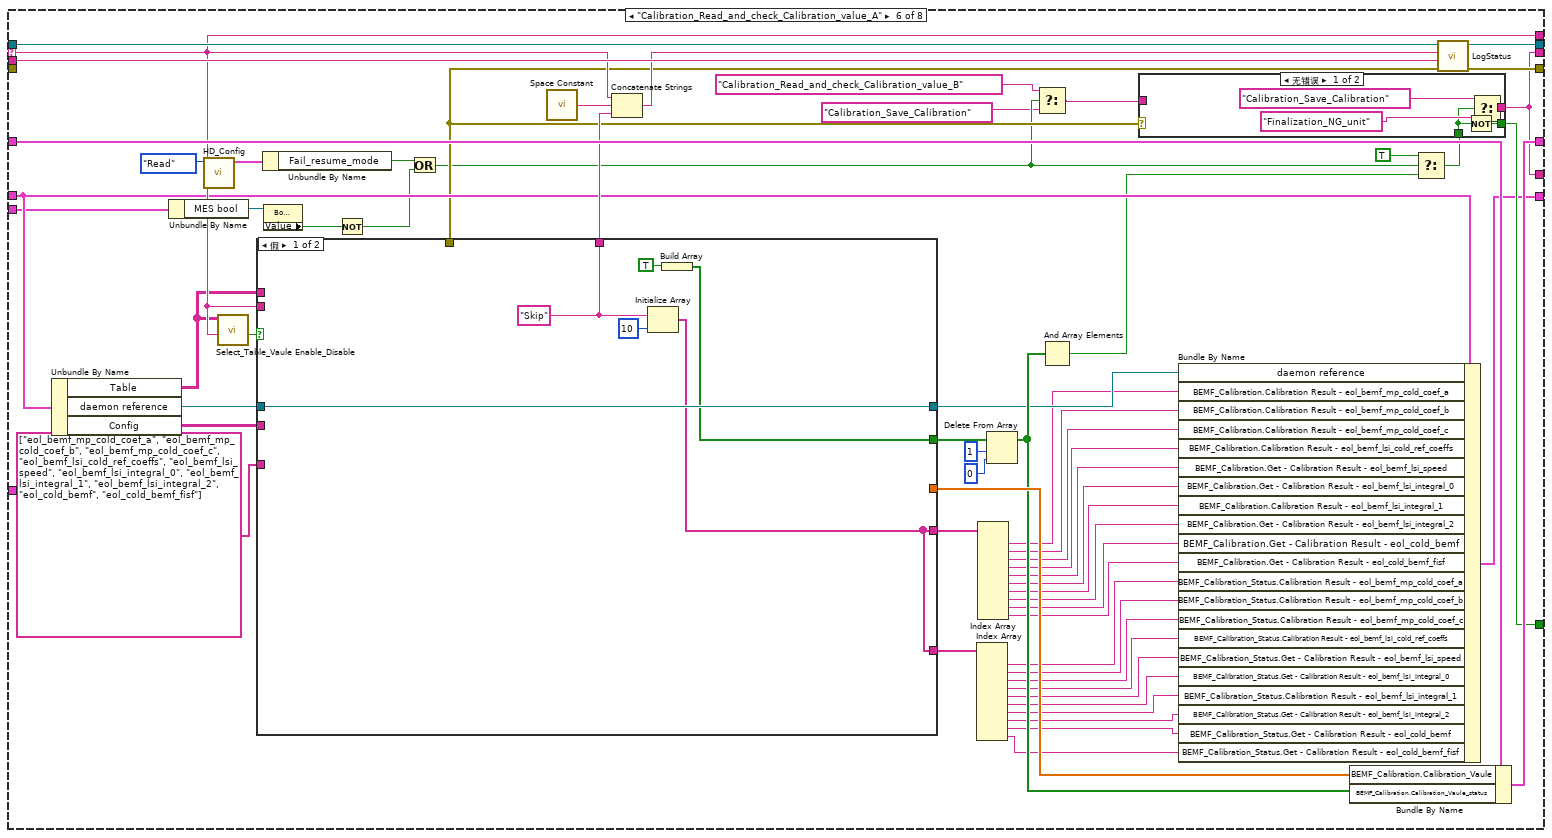
[diagram p17: hidden frame]
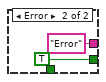
[diagram p18: hidden frame]
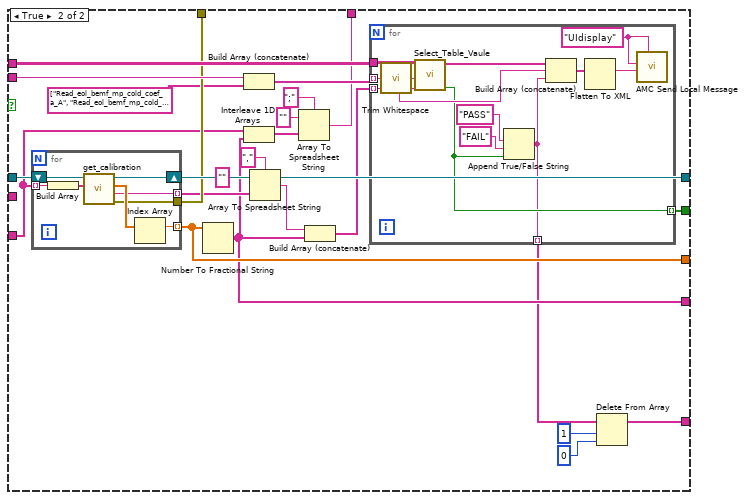
[diagram p19: hidden frame]
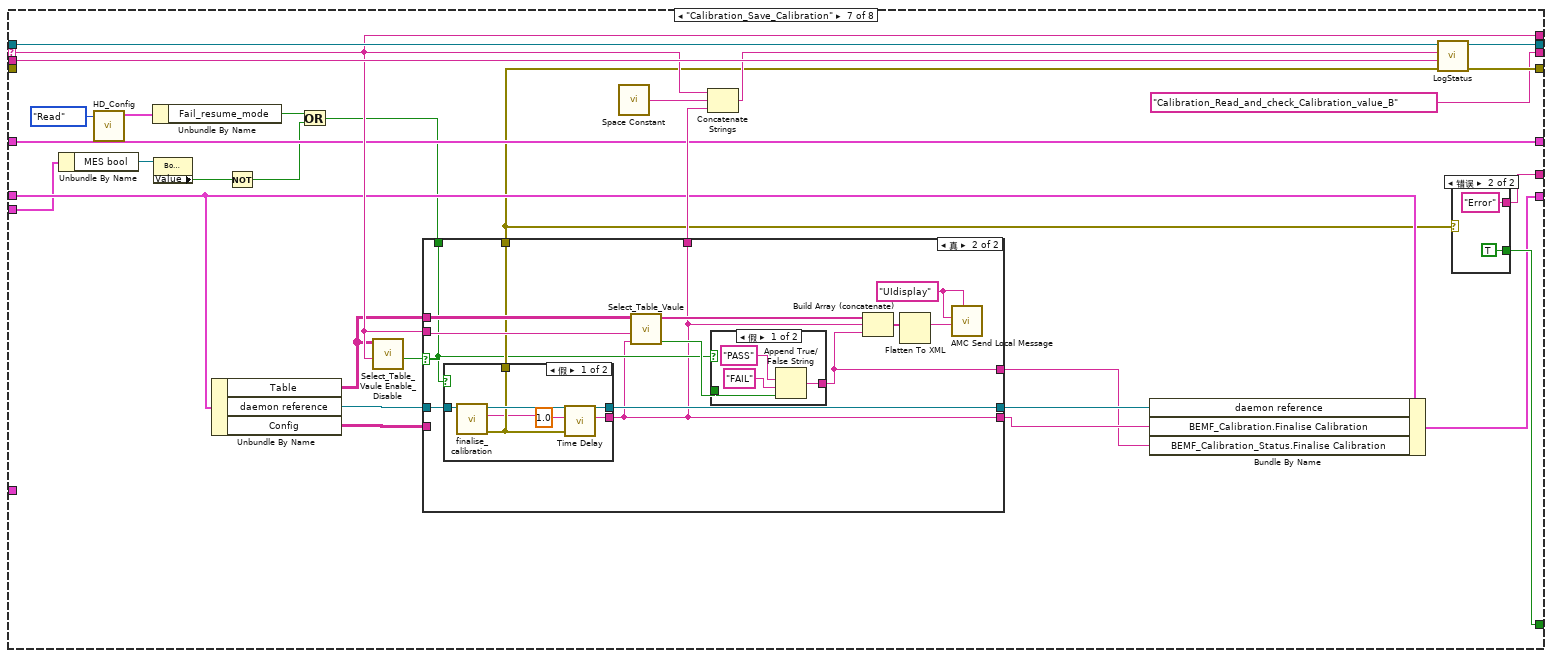
[diagram p20: hidden frame]
diagram:
  n1 = Flush Queue(queue="Message Queue out") -> (queue out=w6:T4)  [unwired: 1 in, 2 out]
  n2 = call "HD_Config.vi"("Step"=enum16{"Initial", "Write", "Read"}."Read") -> ("HD Config out"=w8:T5)  [unwired: 9 in, 1 out]
  n3 = call "AMC Send Local Message.vi"("error in (no error)"="error in (no error)", "Message Name"="Calibration_Read_and_check_DDM_ambient_temperature", "Message Queue in"=w6) -> ("error out"=w13:errorcluster, "Message Queue out"=w14:T4)  [unwired: 7 in]
  n4 = while {
    tunnel: w14 -> [w47]
    tunnel: [w43] -> w5
    tunnel: w13 -> [w41]
    tunnel: [w38] -> w4
    shift-right: [w34] -> w10
    shift-left: "?" -> [w35]
    tunnel: w8 -> [w33]
    tunnel: [w29] -> w7
    shift-right: [w21] -> w2
    shift-left: "Data in" -> [w22]
    tunnel: "AllControls In" -> [w20]
    stop <- w23 stop-if-true
    n5 = Wait (ms)(milliseconds to wait=u32 1 ("等待时间（毫秒）")) -> ()  [unwired: 1 out]
    n6 = call "AMC Read Next Message.vi"("error in (no error)"=w41, "timeout (1ms)"=100, "Message Queue in"=w47) -> ("error out"=w40:errorcluster, "Message Value"=w31:string, "Message Name"=w45:string, "Message Queue out"=w46:T4)  [unwired: 1 in, 4 out]
    n7 = case shown="\"Calibration_Start_Calibration\"" w45 {
      selector: w45 -> [_ w64 w117 w180 w250 w335 w423 w489]
      tunnel: w46 -> [w51 w74 w123 w186 w256 w344 w430 w497]
      tunnel: [w51 w74 w123 w186 w256 w344 w430 w497] -> w44
      tunnel: w40 -> [w50 _ _ w185 _ _ _ _]
      tunnel: [w50 w73 w122 w184 w255 w343 w429 w496] -> w39
      tunnel: [_ w58 w113 w159 w246 w325 w418 TRUE] -> w24
      tunnel: w35 -> [w49 w70 w109 w157 w239 w340 w416 w494]
      tunnel: [w49 w69 w109 w157 w239 w339 w416 w493] -> w34
      tunnel: w31 -> [_ w72 w121 w183 w254 w342 w428 w495]
      tunnel: [_ w64 w117 w180 w250 w335 w423 w489] -> w30
      tunnel: w33 -> [_ _ _ w173 _ _ _ _]
      tunnel: [_ w61 "Calibration_Orifice_Size" "Calibration_Start_Calibration" w245 w331 "Calibration_Read_and_check_Calibration_value_B" w487] -> w32
      tunnel: [_ w61 w114 w155 w245 w331 w419 w487] -> w29
      tunnel: w22 -> [w48 w57 w108 w154 w242 w324 w415 w469]
      tunnel: [w48 w54 w105 w156 w240 w320 w412 w468] -> w21
      tunnel: w20 -> [_ _ _ _ w230 w312 w403 w470]
      frame "假", Default {
      }
      frame "Calibration_Read_and_check_DDM_ambient_temperature" {
        n8 = Unbundle By Name(w57) -> ("Table"=w63:string[][], "daemon reference"=w71:refnum<k5>)
        n9 = call "Select_Table_Vaule Enable_Disable.vi"("Action"=w64, "Table"=w63) -> ("Enable"=w65:bool)  [unwired: 8 in, 1 out]
        n10 = case shown="真" w65 {
          tunnel: w71 -> [w82 w94]
          tunnel: [TRUE w85] -> w62
          tunnel: [w82 w93] -> w55
          tunnel: [w81 w86] -> w66
          tunnel: w64 -> [_ w97]
          tunnel: w63 -> [_ w96]
          tunnel: [_ w90] -> w56
          tunnel: [_ w89] -> w60
          tunnel: T6[] ["eol_cold_bemf_temp"] ("Calibration") -> [_ w88]
          tunnel: [w81 w87] -> w52
          tunnel: [w81 w86] -> w53
          frame False {
            w81 = "Skip" ("response")
          }
          frame True {
            w102 = "UIdisplay" ("Process (\"\" - local)")
            n11 = call "get_calibration.vi"("Calibration"=w88, "daemon reference in"=w94) -> ("error out"=w90:errorcluster, "response"=w86:string, "values"=w91:dbl[], "daemon reference out"=w93:refnum<k5>)  [unwired: 5 in, 1 out]
            n12 = Index Array(array=w91) -> (element=w89:dbl)  [unwired: 1 in]
            n13 = call "Select_Table_Vaule.vi"("Vaule"=w86, "Action"=w97, "Table"=w96) -> ("vaule"=w95:string[])  [unwired: 7 in, 1 out]
            n14 = Equal?(x=w89, y=-1.0) -> (x = y?=w85:bool)
            n15 = Append True/False String(1:TRUE ("选择器"), 2:"FAIL" ("真字符串"), 3:"PASS" ("真字符串")) -> (0:w87:string)  [unwired: 1 in]
            n16 = Build Array (concatenate)(w95, w86, w87) -> (w101:string[])
            n17 = Flatten To XML(anything=w101) -> (xml string=w100:string)
            n18 = call "AMC Send Local Message.vi"("Process (\"\" - local)"=w102, "Message Value"=w100, "Message Name"=w102) -> ()  [unwired: 7 in, 2 out]
          }
        }
        n19 = call <vilib>:"Space Constant.vi"() -> ("String"=w68:string)
        n20 = Concatenate Strings(w64, w68, w66) -> (w67:string)
        n21 = case shown="无错误" w56 {
          tunnel: w62 -> [w75 _]
          tunnel: [w76 "Error" ("Message Name")] -> w61
          tunnel: [_ TRUE] -> w58
          frame No Error {
            n22 = Select(t="Calibration_Set_ambient_temperature_to_DDM", s=w75, f="Calibration_Read_and_check_Calibration_value_A") -> (s? t:f=w76:string)
          }
          frame Error {
          }
        }
        n23 = Bundle By Name(cluster=w57, "daemon reference"=w55, "BEMF_Calibration.Calibration Result - eol_cold_bemf_temp"=w53, "BEMF_Calibration_Status.Calibration Result - eol_cold_bemf_temp"=w52) -> (w54:T2)
        n24 = Bundle By Name(cluster=w70, "BEMF_Calibration.Read_ambient_temperature"=w60) -> (w69:T3)
        n25 = call "LogStatus.vi"("error in (no error)"=w56, "last message"=w72, "message"=w67) -> ("error  out"=w73:errorcluster)  [unwired: 8 in]
      }
      frame "Calibration_Set_ambient_temperature_to_DDM" {
        n26 = Unbundle By Name(w109) -> ("Initialisation.Get_Tester_Parameter"=w116:dbl[])
        n27 = Unbundle By Name(w108) -> ("Table"=w111:string[][], "daemon reference"=w110:refnum<k5>)
        n28 = call "Select_Table_Vaule Enable_Disable.vi"("Action"=w117, "Table"=w111) -> ("Enable"=w118:bool)  [unwired: 8 in, 1 out]
        n29 = case shown="假" w118 {
          tunnel: w110 -> [w127 w141]
          tunnel: [TRUE w143] -> _
          tunnel: [w127 w142] -> w106
          tunnel: [w126 w132] -> w112
          tunnel: w117 -> [_ w146]
          tunnel: w111 -> [_ w145]
          tunnel: w116 -> [_ w139]
          tunnel: [_ w133] -> w107
          tunnel: [_ w132] -> _
          tunnel: [w126 w131] -> w103
          tunnel: [w126 w129] -> w104
          frame False {
            w126 = "Skip" ("response")
          }
          frame True {
            w151 = "UIdisplay" ("Process (\"\" - local)")
            n30 = Index Array(array=w139, index=4 ("索引")) -> (element=w137:dbl)
            n31 = Multiply(x=w137, y=1000.0) -> (x*y=w130:dbl)
            n32 = Build Array(w130) -> (w136:dbl[])
            n33 = call "set_calibration.vi"("values"=w136, "calibration"=T6[] ["eol_cold_bemf_temp"], "daemon reference in"=w141) -> ("error out"=w134:errorcluster, "response"=w132:string, "daemon reference out"=w142:refnum<k5>)  [unwired: 5 in, 1 out]
            n34 = call "Time Delay4"("error in (no error)"=w134) -> ("error out"=w133:errorcluster)  [unwired: 10 in]
            n35 = Number To Decimal String(number=w130) -> (decimal integer string=w129:string)  [unwired: 1 in]
            n36 = call "Select_Table_Vaule.vi"("Vaule"=w132, "Action"=w146, "Table"=w145) -> ("Result"=w143:bool, "vaule"=w144:string[])  [unwired: 7 in]
            n37 = Append True/False String(1:w143, 2:"FAIL" ("真字符串"), 3:"PASS" ("真字符串")) -> (0:w131:string)  [unwired: 1 in]
            n38 = Build Array (concatenate)(w144, w132, w131) -> (w150:string[])
            n39 = Flatten To XML(anything=w150) -> (xml string=w149:string)
            n40 = call "AMC Send Local Message.vi"("Process (\"\" - local)"=w151, "Message Value"=w149, "Message Name"=w151) -> ()  [unwired: 7 in, 2 out]
          }
        }
        n41 = call <vilib>:"Space Constant.vi"() -> ("String"=w120:string)
        n42 = Concatenate Strings(w117, w120, w112) -> (w119:string)
        n43 = Bundle By Name(cluster=w108, "daemon reference"=w106, "BEMF_Calibration.DDM Ambient Temp"=w104, "BEMF_Calibration_Status.DDM Ambient Temp"=w103) -> (w105:T2)
        n44 = call "LogStatus.vi"("error in (no error)"=w107, "last message"=w121, "message"=w119) -> ("error  out"=w122:errorcluster)  [unwired: 8 in]
        n45 = case shown="错误" w107 {
          tunnel: [_ TRUE] -> w113
          tunnel: [_ "Error"] -> w114
          frame No Error {
          }
          frame Error {
          }
        }
      }
      frame "Calibration_Orifice_Size" {
        n46 = Unbundle By Name(w173) -> ("Motor.COM"=w172:refnum<visa-resource-name>)
        n47 = Unbundle By Name(w154) -> ("Config"=w171:string[][])
        n48 = call "Position_Config.vi"("Step"=enum16{"Initial", "Write", "Read"}."Read") -> ("Position Config out"=w168:T8)  [unwired: 9 in, 1 out]
        n49 = call "Index_Config.vi"("Action"="Calibrate_BEMF_Orifice_size", "config"=w171) -> ("data"=w153:string)  [unwired: 9 in]
        n50 = case shown="\"12.7\", 默认" w153 {
          tunnel: w168 -> [w190 w192 w194 w196]
          tunnel: [w189 w191 w193 w195] -> w167
          frame "12.7", Default {
            n51 = Unbundle By Name(w190) -> ("OrificeSize_12.7"=w189:i32)
          }
          frame "13" {
            n52 = Unbundle By Name(w192) -> ("OrificeSize_13"=w191:i32)
          }
          frame "30" {
            n53 = Unbundle By Name(w194) -> ("OrificeSize_30"=w193:i32)
          }
          frame "16" {
            n54 = Unbundle By Name(w196) -> ("OrificeSize_16"=w195:i32)
          }
        }
        n55 = call "IO.vi"("DO DATA"=bool[] [FALSE] ("Writel_IO"), "IO Name"=string[] ["Orifice_fixed_Cylinder"], "IO?"=enum16{"DI", "DO"}."DO") -> ("error out"=w166:errorcluster)  [unwired: 6 in, 2 out]
        n56 = To Long Integer(number=w167) -> (32bit integer=w175:i32)
        n57 = call "Time Delay2"("error in (no error)"=w166) -> ("error out"=w162:errorcluster)  [unwired: 10 in]
        n58 = call "Pulse.vi"("Pulse"=w175) -> ("Pulse"=w176:string)  [unwired: 10 in]
        n59 = call "Motor Visa.vi"("错误输入（无错误）"=w162, "Command"=w176, "VISA资源名称"=w172) -> ("错误输出"=w177:errorcluster, "VISA资源名称输出"=w178:refnum<visa-resource-name>)  [unwired: 6 in, 1 out]
        n60 = call "ABS.vi"() -> ("绝对模式"=w174:string)  [unwired: 11 in]
        n61 = call "Motor Visa.vi"("错误输入（无错误）"=w177, "Command"=w174, "VISA资源名称"=w178) -> ("VISA资源名称输出"=w161:refnum<visa-resource-name>)  [unwired: 6 in, 2 out]
        n62 = while {
          tunnel: w161 -> [w226]
          tunnel: [w211] -> w160
          tunnel: [w205] -> w158
          stop <- w216 stop-if-true
          n63 = call "Get Status.vi"() -> ("Command"=w227:string)  [unwired: 11 in]
          n64 = call "Get Alarm  Error Status.vi"() -> ("AlarmStatus"=w219:string, "ErrorStatus"=w220:string)  [unwired: 10 in]
          n65 = call "Motor Visa.vi"("Command"=w227, "VISA资源名称"=w226) -> ("读取缓冲区"=w225:string, "VISA资源名称输出"=w218:refnum<visa-resource-name>)  [unwired: 7 in, 1 out]
          n66 = Wait (ms)(milliseconds to wait=u32 50 ("等待时间（毫秒）")) -> ()  [unwired: 1 out]
          n67 = call "Motor Visa.vi"("Command"=w220, "VISA资源名称"=w218) -> ("读取缓冲区"=w222:string, "VISA资源名称输出"=w223:refnum<visa-resource-name>)  [unwired: 7 in, 1 out]
          n68 = call "Motor Visa.vi"("Command"=w219, "VISA资源名称"=w223) -> ("读取缓冲区"=w221:string)  [unwired: 7 in, 2 out]
          n69 = call "6-AlarmStatus.vi"("Step"=enum16{"Initial", "Write", "Read"}."Read") -> ("AlarmValue Out"=w209:bool[])  [unwired: 9 in, 1 out]
          n70 = call "Exit.vi"("Step"=enum16{"Initial", "Write", "Read"}."Read" ("step")) -> ("Exit Out"=w207:bool)  [unwired: 9 in, 1 out]
          n71 = call "Stop.vi"("Step"=enum16{"Initial", "Write", "Read"}."Read") -> ("Stop Out"=w206:bool)  [unwired: 9 in, 1 out]
          n72 = call "Alarm and Error Result.vi"("Command"=w221) -> ("Alarm or Error"=w213:bool)  [unwired: 10 in]
          n73 = call "Alarm and Error Result.vi"("Command"=w222) -> ("Alarm or Error"=w212:bool)  [unwired: 10 in]
          n74 = call "Motion Down.vi"("Command"=w225) -> ("Motion Down"=w217:bool)  [unwired: 10 in]
          n75 = Or Array Elements(Boolean array=w209) -> (logical OR=w208:bool)
          n76 = Compound Arithmetic op=OR(w208, w207, w206, w213, w212, w217) -> (w216:bool)
          n77 = Or(x=w213, y=w212) -> (x .or. y?=w211:bool)
          n78 = Compound Arithmetic op=OR(w208, w207, w206) -> (w205:bool)
        }
        n79 = call <vilib>:"Space Constant.vi"() -> ("String"=w182:string)
        n80 = Concatenate Strings(w180, w182, w153) -> (w181:string)
        n81 = Or(x=w158, y=w160) -> (x .or. y?=w159:bool)
        n82 = case shown="真" w158 {
          tunnel: w161 -> [_ w187]
          frame False {
          }
          frame True {
            n83 = call "Stop Command.vi"() -> ("Stop"=w188:string)  [unwired: 11 in]
            n84 = call "Motor Visa.vi"("Command"=w188, "VISA资源名称"=w187) -> ()  [unwired: 7 in, 3 out]
          }
        }
        n85 = case shown="假" w160 {
          tunnel: [_ "Error" ("Message Name")] -> w155
          frame False {
            n86 = call "IO.vi"("DO DATA"=bool[] [TRUE] ("Writel_IO"), "IO Name"=string[] ["Orifice_fixed_Cylinder"], "IO?"=enum16{"DI", "DO"}."DO") -> ("error out"=w200:errorcluster)  [unwired: 6 in, 2 out]
            n87 = call "Time Delay3"("error in (no error)"=w200) -> ()  [unwired: 10 in, 1 out]
          }
          frame True {
            n88 = call "6-AlarmStatus.vi"("AlarmValue"=TRUE, "AlarmIndex"=AlarmIndex."Motor Error", "Step"=enum16{"Initial", "Write", "Read"}."Write") -> ()  [unwired: 7 in, 2 out]
          }
        }
        n89 = Bundle By Name(cluster=w154, "BEMF_Calibration.Restriction Plate Diameter"=w153, "BEMF_Calibration_Status.Restriction Plate Diameter"="PASS") -> (w156:T2)
        n90 = call "LogStatus.vi"("error in (no error)"=w185, "last message"=w183, "message"=w181) -> ("error  out"=w184:errorcluster)  [unwired: 8 in]
      }
      frame "Calibration_Start_Calibration" {
        n91 = Unbundle By Name(w242) -> ("Table"=w249:string[][], "daemon reference"=w253:refnum<k5>, "Config"=w247:string[][])
        n92 = call "Select_Table_Vaule Enable_Disable.vi"("Action"=w250, "Table"=w249) -> ("Enable"=w248:bool)  [unwired: 8 in, 1 out]
        n93 = case shown="真" w248 {
          tunnel: w253 -> [w264 w283]
          tunnel: [w264 w282] -> w241
          tunnel: ["Disable" ("software string") w266] -> w243
          tunnel: w250 -> [_ w268]
          tunnel: w249 -> [_ w281]
          tunnel: w247 -> [_ _]
          tunnel: [TRUE w275] -> w229
          tunnel: [_ w276] -> w244
          tunnel: [_ w266] -> _
          tunnel: [_ w265] -> _
          frame False {
          }
          frame True {
            w274 = "UIdisplay" ("Process (\"\" - local)")
            w279 = u16 0 items=["Both", "LSI", "FISF"] ("calibration type")
            n94 = call "calibrate_bemf.vi"("calibration type"=w279, "calibration wait time ms"=u32 5000, "daemon reference in"=w283) -> ("error out"=w276:errorcluster, "response"=w266:string, "daemon reference out"=w282:refnum<k5>)  [unwired: 5 in, 1 out]
            n95 = Search and Replace String(input string=w266, search string="ERROR" ("搜索字符串")) -> (number of replacements=w277:i32)  [unwired: 6 in, 3 out]
            n96 = Equal To 0?(x=w277) -> (x = 0?=w275:bool)
            n97 = call "Select_Table_Vaule.vi"("Vaule"=w266, "Action"=w268, "Table"=w281) -> ("Result"=w267:bool, "vaule"=w269:string[])  [unwired: 7 in]
            n98 = Append True/False String(1:w267, 2:"FAIL" ("真字符串"), 3:"PASS" ("真字符串")) -> (0:w265:string)  [unwired: 1 in]
            n99 = Build Array (concatenate)(w269, w266, w265) -> (w273:string[])
            n100 = Flatten To XML(anything=w273) -> (xml string=w272:string)
            n101 = call "AMC Send Local Message.vi"("Process (\"\" - local)"=w274, "Message Value"=w272, "Message Name"=w274) -> ()  [unwired: 7 in, 2 out]
          }
        }
        n102 = call <vilib>:"Space Constant.vi"() -> ("String"=w252:string)
        n103 = Concatenate Strings(w250, w252, w243) -> (w251:string)
        n104 = Bundle By Name(cluster=w242, "daemon reference"=w241) -> (w240:T2)
        n105 = Unbundle By Name(w230) -> ("MES bool"=w235:refnum<vi>)
        n106 = call "HD_Config.vi"("Step"=enum16{"Initial", "Write", "Read"}."Read") -> ("HD Config out"=w234:T5)  [unwired: 9 in, 1 out]
        n107 = Unbundle By Name(w234) -> ("Fail_resume_mode"=w236:bool)
        n108 = property class="Bool (严格)"(reference=w235) -> ("Value"=w237:bool)  [unwired: 1 in, 2 out]
        n109 = Not(x=w237) -> (.not. x?=w238:bool)
        n110 = Or(x=w236, y=w238) -> (x .or. y?=w231:bool)
        n111 = Select(t=TRUE, s=w231, f=w229) -> (s? t:f=w228:bool)
        n112 = case shown="无错误" w244 {
          tunnel: [w258 "Error"] -> w245
          tunnel: w228 -> [w257 _]
          frame No Error {
            n113 = Select(t="Calibration_Read_and_check_Calibration_value_A", s=w257, f="Finalization_NG_unit") -> (s? t:f=w258:string)
          }
          frame Error {
          }
        }
        n114 = Not(x=w228) -> (.not. x?=w246:bool)
        n115 = call "LogStatus.vi"("error in (no error)"=w244, "last message"=w254, "message"=w251) -> ("error  out"=w255:errorcluster)  [unwired: 8 in]
      }
      frame "Calibration_Read_and_check_Calibration_value_A" {
        n116 = Unbundle By Name(w324) -> ("Table"=w334:string[][], "daemon reference"=w341:refnum<k5>, "Config"=w332:string[][])
        n117 = Unbundle By Name(w312) -> ("MES bool"=w315:refnum<vi>)
        n118 = call "HD_Config.vi"("Step"=enum16{"Initial", "Write", "Read"}."Read") -> ("HD Config out"=w314:T5)  [unwired: 9 in, 1 out]
        n119 = call "Select_Table_Vaule Enable_Disable.vi"("Action"=w335, "Table"=w334) -> ("Enable"=w333:bool)  [unwired: 8 in, 1 out]
        n120 = case shown="假" w333 {
          tunnel: w341 -> [w357 w380]
          tunnel: [w357 w379] -> w321
          tunnel: [w354 w372] -> w336
          tunnel: w335 -> [_ w376]
          tunnel: w334 -> [_ w381]
          tunnel: w332 -> [_ _]
          tunnel: [w355 w370] -> w305
          tunnel: [_ w378] -> w330
          tunnel: [_ w371] -> w323
          tunnel: T6[] ["eol_bemf_mp_cold_coef_a", "eol_bemf_mp_cold_coef_b", "eol_bemf_mp_cold_coef_c", "eol_bemf_lsi_cold_ref_coeffs", "eol_bemf_lsi_speed", "eol_bemf_lsi_integral_0", "eol_bemf_lsi_integral_1", "eol_bemf_lsi_integral_2", "eol_cold_bemf", "eol_cold_bemf_fisf"] ("Calibration") -> [_ w368]
          tunnel: [w352 w362] -> w322
          tunnel: [w352 w358] -> w294
          frame False {
            w354 = "Skip" ("software string")
            n121 = Initialize Array(w354, 10 ("维数大小")) -> (w352:string[])
            n122 = Build Array(TRUE) -> (w355:bool[])
          }
          frame True {
            n123 = for {
              tunnel: [w382] -> w378 mode=indexing
              tunnel: [w386] -> w371
              tunnel: w368 -> [w385] mode=indexing
              tunnel: [w384] -> w367 mode=indexing
              shift-right: [w388] -> w379
              shift-left: w380 -> [w389]
              n124 = Build Array(w385) -> (w383:T6[])
              n125 = call "get_calibration.vi"("Calibration"=w383, "daemon reference in"=w389) -> ("error out"=w386:errorcluster, "response"=w384:string, "values"=w387:dbl[], "daemon reference out"=w388:refnum<k5>)  [unwired: 5 in, 1 out]
              n126 = Index Array(array=w387) -> (element=w382:dbl)  [unwired: 1 in]
            }
            n127 = Number To Fractional String(number=w378) -> (F-format string=w362:string[])  [unwired: 3 in]
            n128 = Build Array (concatenate)(w376, string[] ["Read_eol_bemf_mp_cold_coef_a_A", "Read_eol_bemf_mp_cold_coef_b_A", "Read_eol_bemf_mp_cold_coef_c_A", "Read_eol_bemf_lsi_cold_ref_coeffs_A", "Read_eol_bemf_lsi_speed_A", "Read_eol_bemf_lsi_integral_0_A", "Read_eol_bemf_lsi_integral_1_A", "Read_eol_bemf_lsi_integral_2_A", "Read_eol_cold_bemf_A", "Read_eol_cold_bemf_fisf_A"]) -> (w377:string[])
            n129 = Interleave 1D Arrays(w368, w362) -> (w375:T6[])
            n130 = Array To Spreadsheet String(delimiter (Tab)=",", array=w367, 3:"" ("format string")) -> (spreadsheet string=w366:string)
            n131 = Array To Spreadsheet String(delimiter (Tab)=";" ("分隔符(Tab)"), array=w375, 3:"" ("格式字符串")) -> (spreadsheet string=w372:string)
            n132 = Build Array (concatenate)(w366, w362) -> (w369:string[])
            n133 = for {
              tunnel: w377 -> [w396] mode=indexing
              tunnel: w381 -> [w395]
              tunnel: w369 -> [w393] mode=indexing
              tunnel: [w392] -> w370 mode=indexing
              tunnel: [w390] -> w359 mode=indexing
              w401 = "UIdisplay" ("Process (\"\" - local)")
              n134 = call <vilib>:"Trim Whitespace.vi"("string"=w396) -> ("trimmed string"=w391:string)  [unwired: 1 in]
              n135 = call "Select_Table_Vaule.vi"("Vaule"=w393, "Action"=w391, "Table"=w395) -> ("Result"=w392:bool, "vaule"=w394:string[])  [unwired: 7 in]
              n136 = Append True/False String(1:w392, 2:"FAIL" ("真字符串"), 3:"PASS" ("真字符串")) -> (0:w390:string)  [unwired: 1 in]
              n137 = Build Array (concatenate)(w394, w393, w390) -> (w400:string[])
              n138 = Flatten To XML(anything=w400) -> (xml string=w399:string)
              n139 = call "AMC Send Local Message.vi"("Process (\"\" - local)"=w401, "Message Value"=w399, "Message Name"=w401) -> ()  [unwired: 7 in, 2 out]
            }
            n140 = Delete From Array(array=w359, length=1 ("长度"), index=0 ("索引")) -> (array with subset deleted=w358:string[])  [unwired: 1 out]
          }
        }
        n141 = Unbundle By Name(w314) -> ("Fail_resume_mode"=w316:bool)
        n142 = property class="Bool (严格)"(reference=w315) -> ("Value"=w317:bool)  [unwired: 1 in, 2 out]
        n143 = Not(x=w317) -> (.not. x?=w318:bool)
        n144 = Or(x=w316, y=w318) -> (x .or. y?=w309:bool)
        n145 = call <vilib>:"Space Constant.vi"() -> ("String"=w338:string)
        n146 = Concatenate Strings(w335, w338, w336) -> (w337:string)
        n147 = Index Array(array=w294) -> (element #1=w293:string, element #2=w292:string, element #3=w291:string, element #4=w290:string, element #5=w289:string, element #6=w288:string, element #7=w287:string, element #8=w286:string, element #9=w285:string, element #10=w284:string)  [unwired: 10 in]
        n148 = Index Array(array=w322) -> (element #1=w304:string, element #2=w303:string, element #3=w302:string, element #4=w301:string, element #5=w300:string, element #6=w299:string, element #7=w298:string, element #8=w297:string, element #9=w296:string, element #10=w295:string)  [unwired: 10 in]
        n149 = Delete From Array(array=w305, length=1 ("长度"), index=0 ("索引")) -> (array with subset deleted=w326:bool[])  [unwired: 1 out]
        n150 = Select(t="Calibration_Read_and_check_Calibration_value_B", s=w309, f="Calibration_Save_Calibration") -> (s? t:f=w306:string)
        n151 = And Array Elements(Boolean array=w326) -> (logical AND=w311:bool)
        n152 = Bundle By Name(cluster=w324, "daemon reference"=w321, "BEMF_Calibration.Calibration Result - eol_bemf_mp_cold_coef_a"=w304, "BEMF_Calibration.Calibration Result - eol_bemf_mp_cold_coef_b"=w303, "BEMF_Calibration.Calibration Result - eol_bemf_mp_cold_coef_c"=w302, "BEMF_Calibration.Calibration Result - eol_bemf_lsi_cold_ref_coeffs"=w301, "BEMF_Calibration.Get - Calibration Result - eol_bemf_lsi_speed"=w300, "BEMF_Calibration.Get - Calibration Result - eol_bemf_lsi_integral_0"=w299, "BEMF_Calibration.Calibration Result - eol_bemf_lsi_integral_1"=w298, "BEMF_Calibration.Get - Calibration Result - eol_bemf_lsi_integral_2"=w297, "BEMF_Calibration.Get - Calibration Result - eol_cold_bemf"=w296, "BEMF_Calibration.Get - Calibration Result - eol_cold_bemf_fisf"=w295, "BEMF_Calibration_Status.Calibration Result - eol_bemf_mp_cold_coef_a"=w293, "BEMF_Calibration_Status.Calibration Result - eol_bemf_mp_cold_coef_b"=w292, "BEMF_Calibration_Status.Calibration Result - eol_bemf_mp_cold_coef_c"=w291, "BEMF_Calibration_Status.Calibration Result - eol_bemf_lsi_cold_ref_coeffs"=w290, "BEMF_Calibration_Status.Get - Calibration Result - eol_bemf_lsi_speed"=w289, "BEMF_Calibration_Status.Get - Calibration Result - eol_bemf_lsi_integral_0"=w288, "BEMF_Calibration_Status.Calibration Result - eol_bemf_lsi_integral_1"=w287, "BEMF_Calibration_Status.Get - Calibration Result - eol_bemf_lsi_integral_2"=w286, "BEMF_Calibration_Status.Get - Calibration Result - eol_cold_bemf"=w285, "BEMF_Calibration_Status.Get - Calibration Result - eol_cold_bemf_fisf"=w284) -> (w320:T2)
        n153 = Bundle By Name(cluster=w340, "BEMF_Calibration.Calibration_Vaule"=w330, "BEMF_Calibration.Calibration_Vaule_status"=w326) -> (w339:T3)
        n154 = Select(t=TRUE, s=w309, f=w311) -> (s? t:f=w310:bool)
        n155 = case shown="无错误" w323 {
          tunnel: [w348 "Error"] -> w331
          tunnel: w310 -> [w347 _]
          tunnel: [w346 TRUE] -> w325
          tunnel: w306 -> [_ _]
          frame No Error {
            n156 = Not(x=w347) -> (.not. x?=w346:bool)
            n157 = Select(t="Calibration_Save_Calibration", s=w347, f="Finalization_NG_unit") -> (s? t:f=w348:string)
          }
          frame Error {
          }
        }
        n158 = call "LogStatus.vi"("error in (no error)"=w323, "last message"=w342, "message"=w337) -> ("error  out"=w343:errorcluster)  [unwired: 8 in]
      }
      frame "Calibration_Save_Calibration" {
        n159 = Unbundle By Name(w403) -> ("MES bool"=w406:refnum<vi>)
        n160 = call "HD_Config.vi"("Step"=enum16{"Initial", "Write", "Read"}."Read") -> ("HD Config out"=w405:T5)  [unwired: 9 in, 1 out]
        n161 = Unbundle By Name(w405) -> ("Fail_resume_mode"=w407:bool)
        n162 = property class="Bool (严格)"(reference=w406) -> ("Value"=w408:bool)  [unwired: 1 in, 2 out]
        n163 = Unbundle By Name(w415) -> ("Table"=w422:string[][], "daemon reference"=w427:refnum<k5>, "Config"=w420:string[][])
        n164 = Not(x=w408) -> (.not. x?=w409:bool)
        n165 = Or(x=w407, y=w409) -> (x .or. y?=w402:bool)
        n166 = call "Select_Table_Vaule Enable_Disable.vi"("Action"=w423, "Table"=w422) -> ("Enable"=w421:bool)  [unwired: 8 in, 1 out]
        n167 = case shown="真" w421 {
          tunnel: w427 -> [w434 w444]
          tunnel: [w434 w443] -> w413
          tunnel: [w433 w435] -> w417
          tunnel: w423 -> [_ w442]
          tunnel: w422 -> [_ w441]
          tunnel: w420 -> [_ _]
          tunnel: [_ w438] -> w414
          tunnel: [w433 w435] -> w411
          tunnel: [w433 w437] -> w410
          tunnel: w402 -> [_ w436]
          frame False {
            w433 = "Skip" ("software string")
            (unwired) TRUE
          }
          frame True {
            w447 = "UIdisplay" ("Process (\"\" - local)")
            n168 = case shown="假" w436 {
              tunnel: w444 -> [w457 w459]
              tunnel: [w456 w459] -> w443
              tunnel: [w455 _] -> w438
              tunnel: [w454 "Skip" ("response")] -> w435
              frame False {
                n169 = call "finalise_calibration.vi"("daemon reference in"=w457) -> ("error out"=w455:errorcluster, "response"=w454:string, "daemon reference out"=w456:refnum<k5>)  [unwired: 7 in, 1 out]
                n170 = call "Time Delay"("error in (no error)"=w455, "Delay Time (s)"=1.0) -> ()  [unwired: 9 in, 1 out]
              }
              frame True {
              }
            }
            n171 = call "Select_Table_Vaule.vi"("Vaule"=w435, "Action"=w442, "Table"=w441) -> ("Result"=w439:bool, "vaule"=w440:string[])  [unwired: 7 in]
            n172 = case shown="假" w436 {
              tunnel: w439 -> [w449 _]
              tunnel: [w448 "Skip" ("response")] -> w437
              frame False {
                n173 = Append True/False String(1:w449, 2:"FAIL" ("真字符串"), 3:"PASS" ("真字符串")) -> (0:w448:string)  [unwired: 1 in]
              }
              frame True {
              }
            }
            n174 = Build Array (concatenate)(w440, w435, w437) -> (w446:string[])
            n175 = Flatten To XML(anything=w446) -> (xml string=w445:string)
            n176 = call "AMC Send Local Message.vi"("Process (\"\" - local)"=w447, "Message Value"=w445, "Message Name"=w447) -> ()  [unwired: 7 in, 2 out]
          }
        }
        n177 = call <vilib>:"Space Constant.vi"() -> ("String"=w426:string)
        n178 = Concatenate Strings(w423, w426, w417) -> (w425:string)
        n179 = Bundle By Name(cluster=w415, "daemon reference"=w413, "BEMF_Calibration.Finalise Calibration"=w411, "BEMF_Calibration_Status.Finalise Calibration"=w410) -> (w412:T2)
        n180 = call "LogStatus.vi"("error in (no error)"=w414, "last message"=w428, "message"=w425) -> ("error  out"=w429:errorcluster)  [unwired: 8 in]
        n181 = case shown="错误" w414 {
          tunnel: [_ TRUE] -> w418
          tunnel: [_ "Error"] -> w419
          frame No Error {
          }
          frame Error {
          }
        }
      }
      frame "Calibration_Read_and_check_Calibration_value_B" {
        n182 = Unbundle By Name(w469) -> ("Table"=w482:string[][], "daemon reference"=w481:refnum<k5>)
        n183 = Unbundle By Name(w494) -> ("BEMF_Calibration.Calibration_Vaule"=w483:dbl[])
        n184 = call "Select_Table_Vaule Enable_Disable.vi"("Action"=w489, "Table"=w482) -> ("Enable"=w488:bool)  [unwired: 8 in, 1 out]
        n185 = case shown="假" w488 {
          tunnel: w481 -> [w506 w533]
          tunnel: [w506 w532] -> w464
          tunnel: [w505 w525] -> w490
          tunnel: w489 -> [_ w530]
          tunnel: w482 -> [_ w534]
          tunnel: [_ w515] -> w485
          tunnel: [_ w524] -> w467
          tunnel: T6[] ["eol_cold_bemf", "eol_cold_bemf_fisf"] ("Calibration") -> [_ w523]
          tunnel: w483 -> [_ w518]
          tunnel: [_ w513] -> w466
          tunnel: [w504 w510] -> w465
          tunnel: [_ w508] -> _
          tunnel: [_ w507] -> _
          frame False {
            w505 = "Skip" ("software string")
            n186 = Initialize Array(w505, 3 ("维数大小")) -> (w504:string[])
          }
          frame True {
            n187 = for {
              tunnel: [w535] -> w515 mode=indexing
              tunnel: [w539] -> w524
              tunnel: w523 -> [w538] mode=indexing
              tunnel: [w537] -> w522 mode=indexing
              shift-right: [w541] -> w532
              shift-left: w533 -> [w542]
              n188 = Build Array(w538) -> (w536:T6[])
              n189 = call "get_calibration.vi"("Calibration"=w536, "daemon reference in"=w542) -> ("error out"=w539:errorcluster, "response"=w537:string, "values"=w540:dbl[], "daemon reference out"=w541:refnum<k5>)  [unwired: 5 in, 1 out]
              n190 = Index Array(array=w540) -> (element=w535:dbl)  [unwired: 1 in]
            }
            n191 = Array Subset(array=w518, index=8, length=2) -> (w514:dbl[])
            n192 = Number To Fractional String(number=w515) -> (F-format string=w529:string[])  [unwired: 3 in]
            n193 = Build Array (concatenate)(w530, string[] ["Read_eol_cold_bemf_B", "Read_eol_cold_bemf_fisf_B"]) -> (w531:string[])
            n194 = Interleave 1D Arrays(w523, w529) -> (w528:T6[])
            n195 = Array To Spreadsheet String(delimiter (Tab)=";", array=w522, 3:"" ("format string")) -> (spreadsheet string=w509:string)
            n196 = Array To Spreadsheet String(delimiter (Tab)=";" ("分隔符(Tab)"), array=w528, 3:"" ("格式字符串")) -> (spreadsheet string=w525:string)
            n197 = Build Array (concatenate)(w509, w529) -> (w508:string[])
            n198 = Equal?(x=w515, y=w514) -> (x = y?=w513:bool[])
            n199 = Build Array (concatenate)(TRUE, w513) -> (w511:bool[])
            n200 = for {
              tunnel: w531 -> [w555] mode=indexing
              tunnel: w534 -> [w554]
              tunnel: w508 -> [w552] mode=indexing
              tunnel: w511 -> [w549]
              tunnel: [w547] -> w510 mode=indexing
              tunnel: [w543] -> w507 mode=indexing
              i -> [w548]
              w558 = "UIdisplay" ("Process (\"\" - local)")
              n201 = call <vilib>:"Trim Whitespace.vi"("string"=w555) -> ("trimmed string"=w551:string)  [unwired: 1 in]
              n202 = Equal To 0?(x=w548) -> (x = 0?=w550:bool)
              n203 = call "Select_Table_Vaule.vi"("Vaule"=w552, "Action"=w551, "Table"=w554) -> ("Result"=w544:bool, "vaule"=w553:string[])  [unwired: 7 in]
              n204 = case shown="假" w550 {
                tunnel: w544 -> [_ w566]
                tunnel: [w562 w565] -> w547
                tunnel: w549 -> [w561 _]
                tunnel: w548 -> [w559 _]
                frame False {
                  n205 = Index Array(array=w561, index=w559) -> (element=w560:bool)
                  n206 = Append True/False String(1:w560, 2:"FAIL" ("真字符串"), 3:"PASS" ("真字符串")) -> (0:w562:string)  [unwired: 1 in]
                }
                frame True {
                  n207 = Append True/False String(1:w566, 2:"FAIL" ("真字符串"), 3:"PASS" ("真字符串")) -> (0:w565:string)  [unwired: 1 in]
                }
              }
              n208 = Build Array (concatenate)(w553, w552, w547) -> (w557:string[])
              n209 = Flatten To XML(anything=w557) -> (xml string=w556:string)
              n210 = Append True/False String(1:w544, 2:"FAIL" ("真字符串"), 3:"PASS" ("真字符串")) -> (0:w543:string)  [unwired: 1 in]
              n211 = call "AMC Send Local Message.vi"("Process (\"\" - local)"=w558, "Message Value"=w556, "Message Name"=w558) -> ()  [unwired: 7 in, 2 out]
            }
          }
        }
        n212 = call <vilib>:"Space Constant.vi"() -> ("String"=w492:string)
        n213 = Concatenate Strings(w489, w492, w490) -> (w491:string)
        n214 = Unbundle By Name(w470) -> ("MES bool"=w476:refnum<vi>)
        n215 = call "HD_Config.vi"("Step"=enum16{"Initial", "Write", "Read"}."Read") -> ("HD Config out"=w475:T5)  [unwired: 9 in, 1 out]
        n216 = Unbundle By Name(w475) -> ("Fail_resume_mode"=w477:bool)
        n217 = property class="Bool (严格)"(reference=w476) -> ("Value"=w478:bool)  [unwired: 1 in, 2 out]
        n218 = Not(x=w478) -> (.not. x?=w479:bool)
        n219 = Or(x=w477, y=w479) -> (x .or. y?=w480:bool)
        n220 = And Array Elements(Boolean array=w466) -> (logical AND=w471:bool)
        n221 = Select(t=TRUE, s=w480, f=w471) -> (s? t:f=w472:bool)
        n222 = Index Array(array=w465, index #1=1 ("索引"), index #2=2 ("索引")) -> (element #1=w461:string, element #2=w460:string)
        n223 = case shown="无错误" w467 {
          tunnel: [w499 "Error"] -> w487
          tunnel: w472 -> [w498 _]
          frame No Error {
            n224 = Select(t="Power_Tunings_and_AW_Performance_Test", s=w498, f="Finalization_NG_unit") -> (s? t:f=w499:string)
          }
          frame Error {
          }
        }
        n225 = Bundle By Name(cluster=w469, "daemon reference"=w464, "BEMF_Calibration.Compare -Calibration Result - eol_cold_bemf"=w461, "BEMF_Calibration.Compare -Calibration Result - eol_cold_bemf_fisf"=w460, "BEMF_Calibration_Status.Compare -Calibration Result - eol_cold_bemf"=w461, "BEMF_Calibration_Status.Compare -Calibration Result - eol_cold_bemf_fisf"=w460) -> (w468:T2)
        n226 = Bundle By Name(cluster=w494, "BEMF_Calibration.Calibration_Vaule _B"=w485, "BEMF_Calibration.Calibration_Vaule_B_status"=w466) -> (w493:T3)
        n227 = call "LogStatus.vi"("error in (no error)"=w467, "last message"=w495, "message"=w491) -> ("error  out"=w496:errorcluster)  [unwired: 8 in]
      }
    }
    n228 = call "Stop.vi"("Step"=enum16{"Initial", "Write", "Read"}."Read") -> ("Stop Out"=w26:bool)  [unwired: 9 in, 1 out]
    n229 = call "Exit.vi"("Step"=enum16{"Initial", "Write", "Read"}."Read" ("step")) -> ("Exit Out"=w25:bool)  [unwired: 9 in, 1 out]
    n230 = call "6-AlarmStatus.vi"("Step"=enum16{"Initial", "Write", "Read"}."Read") -> ("AlarmValue Out"=w18:bool[])  [unwired: 9 in, 1 out]
    n231 = Or Array Elements(Boolean array=w18) -> (logical OR=w17:bool)
    n232 = Compound Arithmetic op=OR(w24, w26, w25, w17) -> (w23:bool)
    n233 = call "AMC Run Step.vi"("Message Queue In"=w44, "Message Name"=w32, "Message Value"=w30, "error in (no error)"=w39, "Mli/Sig"=FALSE) -> ("Message Queue Out"=w43:T4, "error out"=w38:errorcluster)  [unwired: 13 in]
  }
  "Message Queue Out" <- w5
  "error out" <- w4
  "Data" <- w10
  "Flow" <- w7
  "Data out" <- w2
